vi "Preset_Manager_Main_Integrated2.0.vi"(4 "Virtual Devices List":string[](array[string]), 6 "Filtered Devices List":string[](array[string]), 8 "Experiment Name":string, 10 "DevStatusQueue":refnum<queue>, 11 "Software Root":string) -> ()   [LabVIEW 2020]
uses:
  <vilib>/Utility/miscctls.llb/LVRowAndColumnTypeDef.ctl
  Shared/MySQL/Preset Query Enum.ctl
  <userlib>/_OpenG.lib/array/array.llb/Delete Elements from 1D Array (String)__ogtk.vi
  <userlib>/_OpenG.lib/array/array.llb/openg_array.lvlib
panel:
  out "Queue Progress Bar":ext(slide) scale=0.0..1.0
  out "Queue Size":i32
  out "Current Preset Queue Element":string
  in  "Expt Devices Not On":i32(listbox)
  in  "Preset Devices Not in Experiment":i32(listbox)
  out "Active Preset":string
  out "Preset Execution Indicator":bool caption="Preset Executed"
  in  "EXIT":bool
  in  "Using Queue":bool
  in  "Tab Control":T1(tab)
  in  "Execute Preset":bool
  in  "Delete Preset":bool
  in  "Save as Preset":bool
  in  "Preset Menu":u16(ring) items=["None", "Pulsed Alignment", "3J", "Diode", "26J", "SingleShot", "1Hz", "800 MAX ND", "Amp3-8J-CapExit", "SDI", "CapInHexPosition", "CapOutHexFiberPosition", "Full Heater, Frog Out", "Full Heater, Frog In", "MagSpecSimulateBoff", "Pulsed", "CW", "Amp2, Clunker In", "Amp3-17J", "MagSpecSimulateBon", "SMFiber-In", "SMFiber-Out", "Amp3-MegaAttenuator", "developer", "developer_main", "developer_test_1", "dev_simcam_2", "dev_simcam_3"]
  in  "Load ECS to Table":bool
  in  "Navigate to ECS File":path
  in  "Preset Table Control":string[][](table)
  in  "Choose Values":bool
  in  "Left Join":bool
  in  "Reset Queue":bool
  in  "Queue Table Control":string[][](table)
  in  "Queue Table":string[][](table)
  in  "Execute Queue":bool
  out "PRESET FROM DB":string[][](table)
  out "ECS File":string[][](table)
  out "Coordinate Array":i32[][](array[numeric])
  out "Devices not started":string[](array[string]) caption="Devices not ready for scan"
  out "Active Device array":bool[](array[boolean])
  out "Active Dev/IP":string[](array[string])
  out "Device Errors":string[][](array[string])
  out "Queue Element":i32
  in  "Poll Count":i32
  in  "Mcast address":string
  in  "MCast Remote":u16
  in  "UDP timeout ms":i32
  in  "MC Multicast":refnum<k16>
  in  "My IP":string
  in  "All Devices Core Info":string[][](array[string])
  out "error out":errorcluster
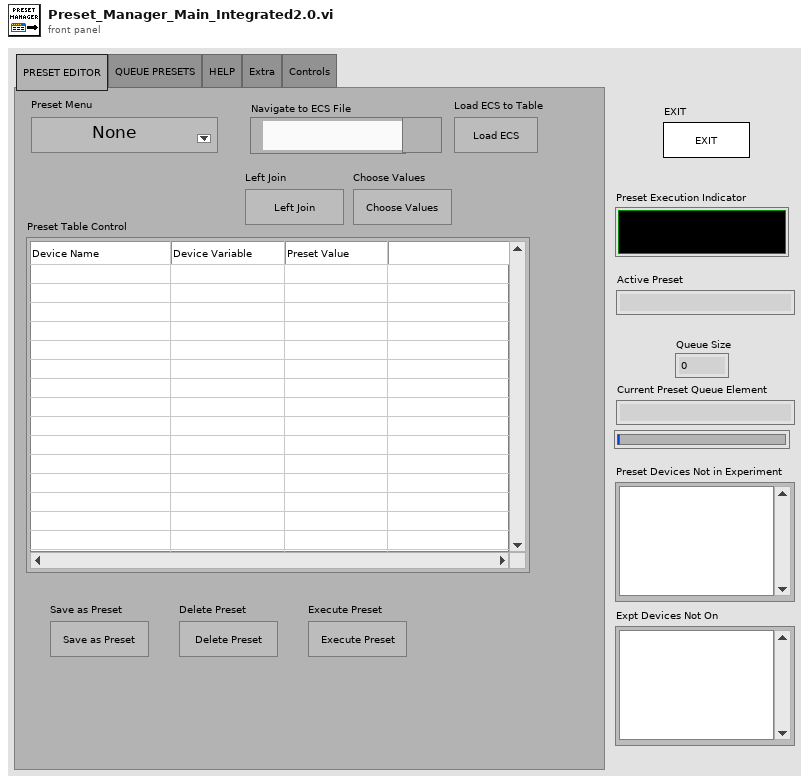
[diagram p1: front panel]
types:
  T1 = enum32{"PRESET EDITOR", "QUEUE PRESETS", "HELP", "Extra", "Controls"}
  T2 = typedef "LVRowAndColumnTypeDef.ctl" = cluster{"Row":i32, "Column":i32}
  T3 = typedef "Preset Query Enum.ctl" = enum16{"Get Locations", "Get all IPs and MACs", "Get classes", "Get expt variables to set at scanstart for particular device", "Get expt devices and variables with start values", "Get expt devices and variables (with data to get)", "Get expt devices with data to get", "Get Expt devices and GUIs", "Get all devices basic properties", "Get Virtual Devices Core Info", "Get Expt names", "Get experiment basic properties", "Get experiment alarm variables", "Get MC Ports", "Get device network comm port", "Get devicetype lvclass path", "Get basic device properties", "Get Init Order", "Get all setable variables of a device", "Get device variable aliases", "Get force values of all settable variables", "Get all variables of a devicetype", "Get all variables of a device", "Get plotter details", "Get Saved Scans", "Get Scan Info", "GetGeneralGUIs", "Get expt for plotter", "Get plotter IDs from expt", "Get all devices", "Get all Virtual Devices", "Get all aliases", "Get variable and device info for Virtual Device", "GetItemLocatorIP", "Get IPs for GUIs", "Get DeviceType from Device", "GetLocalPortRange", "GetDevicePresetVariables", "Get Device Configuration", "GetAllPresetNames", "GetAllConfigurationNames", "GetPresetDeviceNames", "GetDeviceAliases", "GetDevicesOfClass"}
  T4 = enum32{"Invalid", "Standard", "Closed", "Hidden", "Minimized", "Maximized"}
  T5 = enum32{"invalid app kind", "Development System", "Run Time System", "Student Edition", "Embedded LabVIEW", "Evaluation", "Custom"}
  T6 = cluster{"Core":cluster{"Current VI Reference":refnum<vi>, "Close Panel on Exit?":bool}, "Your Boolean data":bool, "String":string, "Preset Table Control":string[][], "Column Headers[]":string[], "Queue Table Control":string[][], "Preset Manager Cluster":cluster{"PresetName":string, "Mcast command":string, "Current Preset Devices":string[], "My IP":string, "Mcast address":string, "Software Root":string, "Experiment Name":string, "MCast Remote":u16, "UDP timeout ms":i32, "MC Multicast":refnum<k16>, "All Devices Core Info":string[][], "Filtered Devices List":string[], "Virtual Devices List":string[], "DevStatusQueue":refnum<queue>}}
  T7 = typedef "LVPoint32TypeDef.ctl" = cluster{"Horizontal":i32, "Vertical":i32}
  T8 = cluster{"Current VI Reference":refnum<vi>, "Close Panel on Exit?":bool}
  T9 = cluster{"PresetName":string, "Mcast command":string, "Current Preset Devices":string[], "My IP":string, "Mcast address":string, "Software Root":string, "Experiment Name":string, "MCast Remote":u16, "UDP timeout ms":i32, "MC Multicast":refnum<k16>, "All Devices Core Info":string[][], "Filtered Devices List":string[], "Virtual Devices List":string[], "DevStatusQueue":refnum<queue>}
  T10 = enum16{"Left Button", "Center Button", "Right Button", "Window Close"}
  T11 = typedef "mysql_authentication.ctl" = cluster{"User":string, "Password":string, "Database":string}
  T12 = cluster{"Port":u16, "IP Address":string, "Authentication":T11}
  T13 = typedef "preset diagnostics.ctl" = cluster{"Active Preset Achieved":bool, "Devices with Active Preset Not Set":string[], "Dev Presets":string[], "All Preset Devices ON?":bool[]}
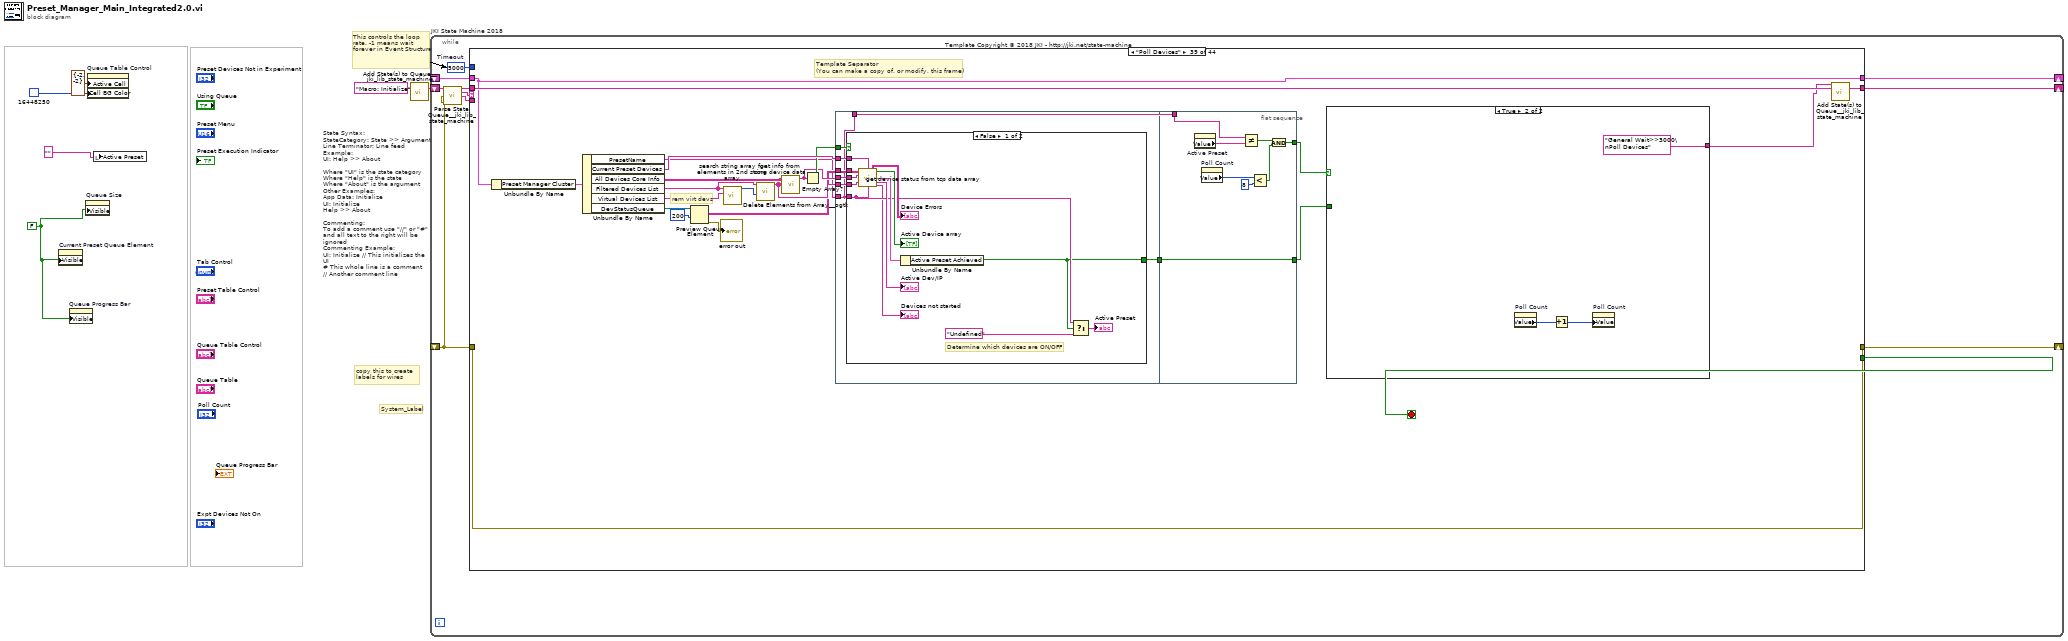
[diagram p0: block diagram]
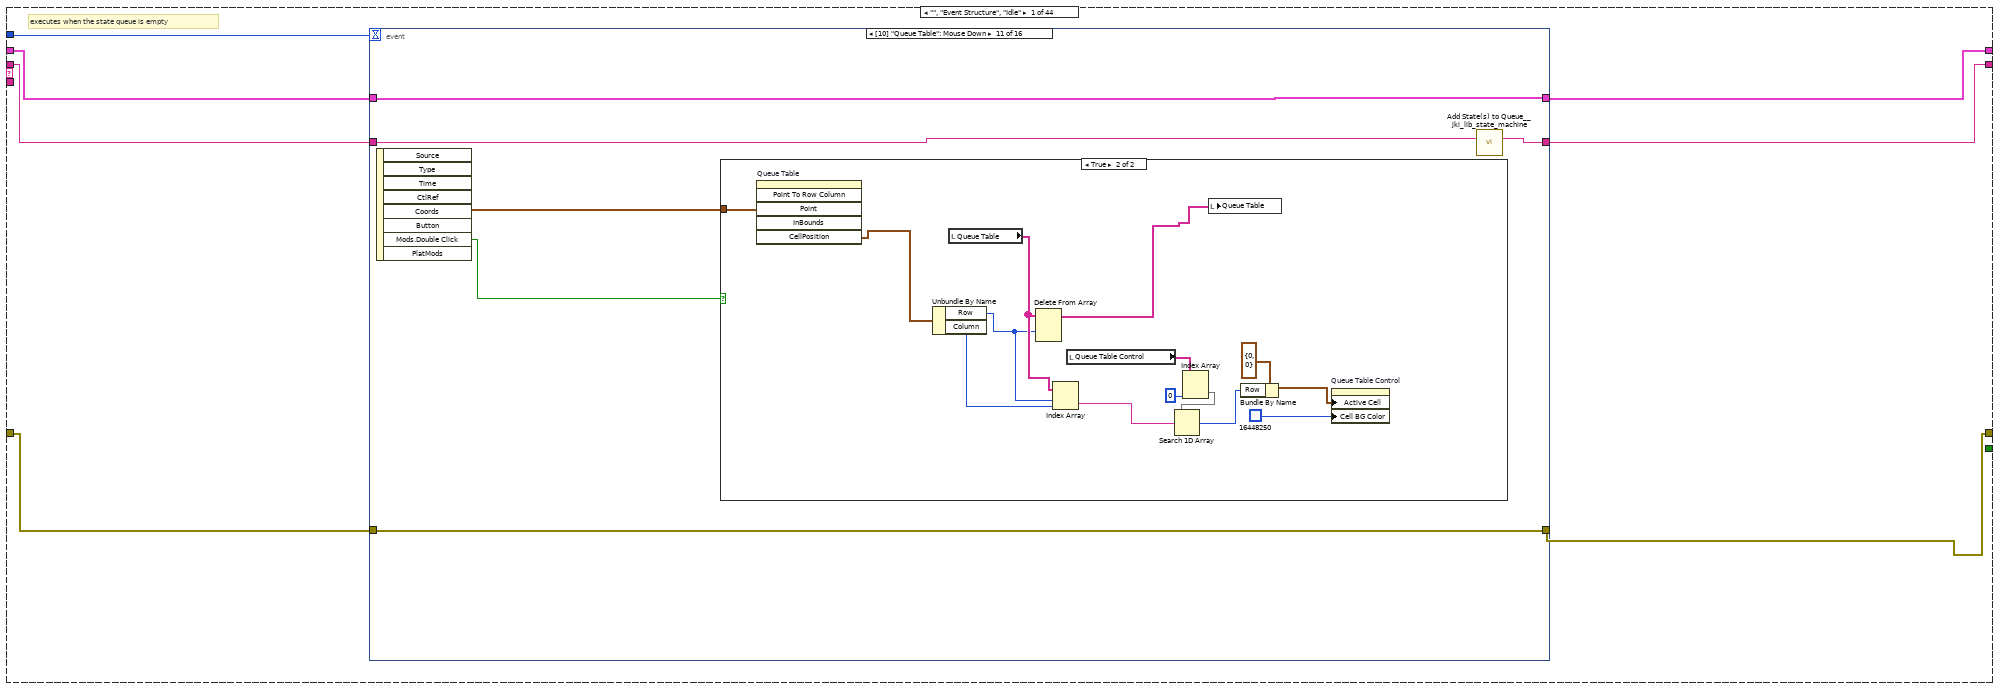
[diagram p2: hidden frame]
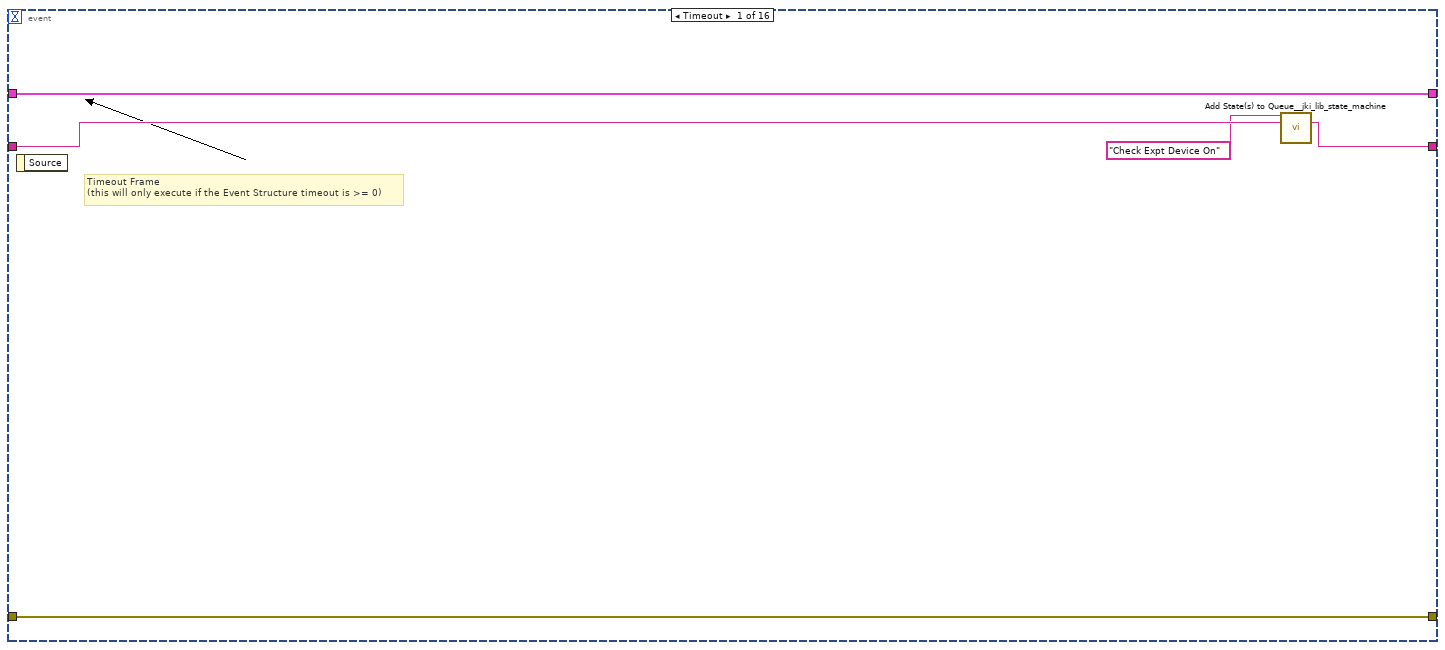
[diagram p3: hidden frame]
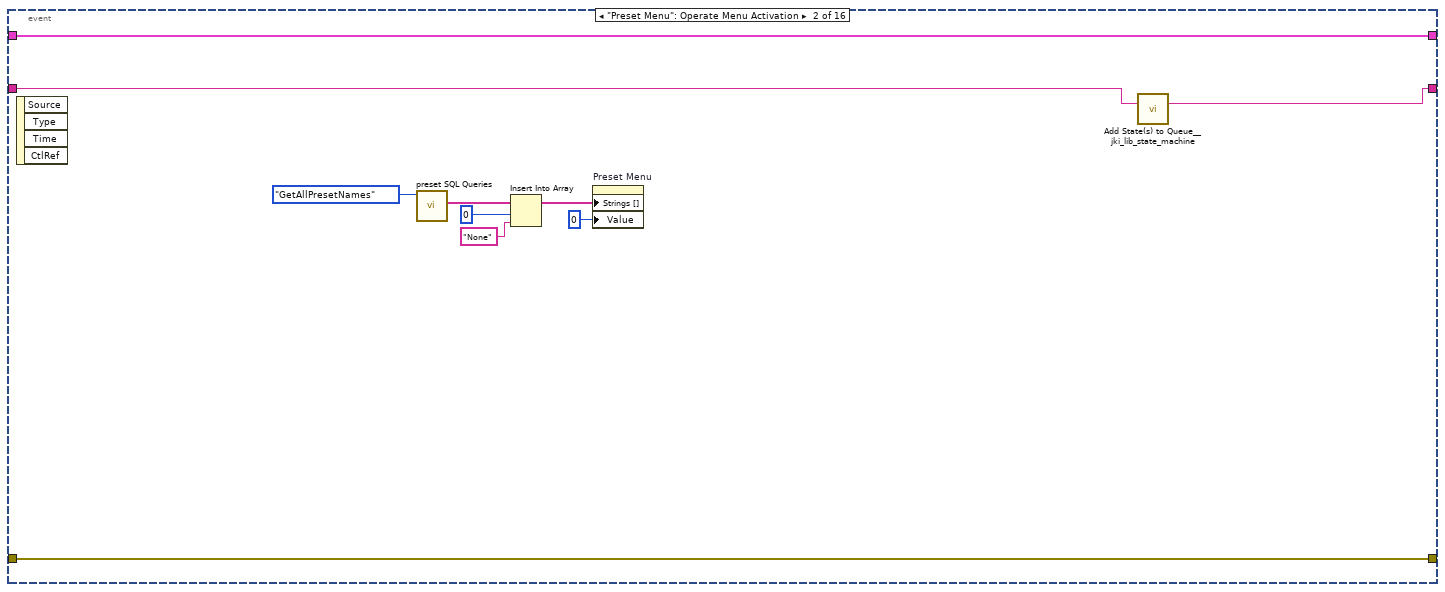
[diagram p4: hidden frame]
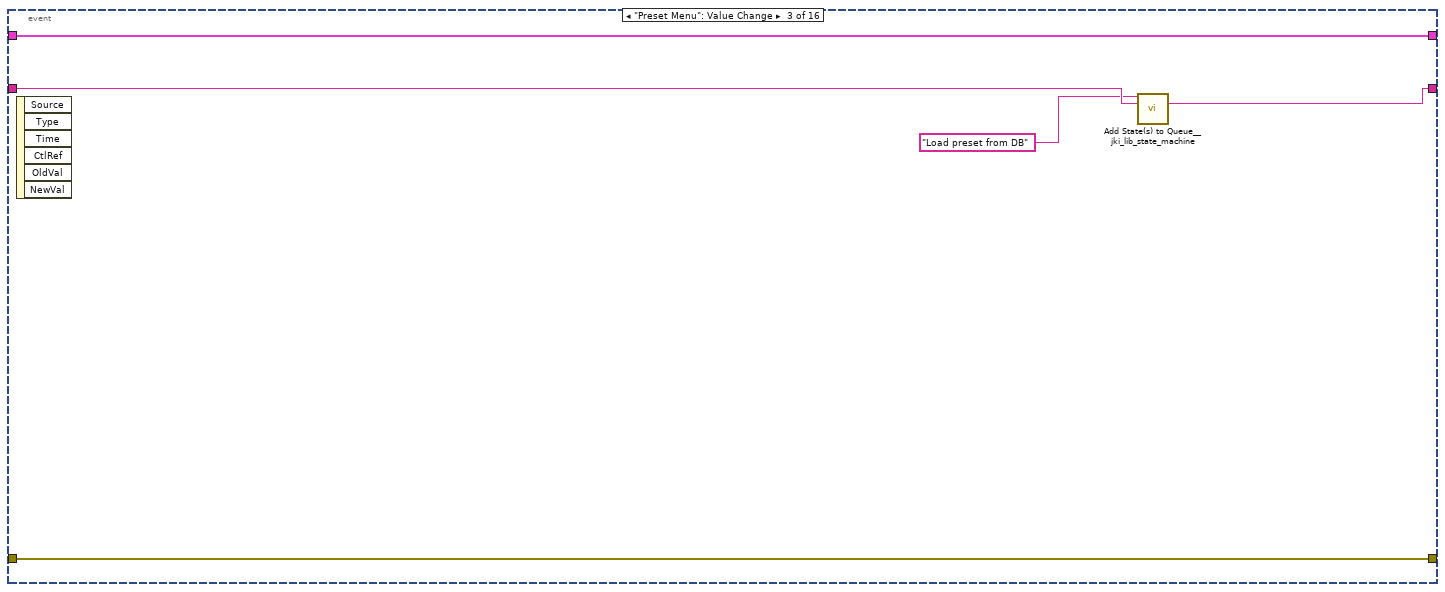
[diagram p5: hidden frame]
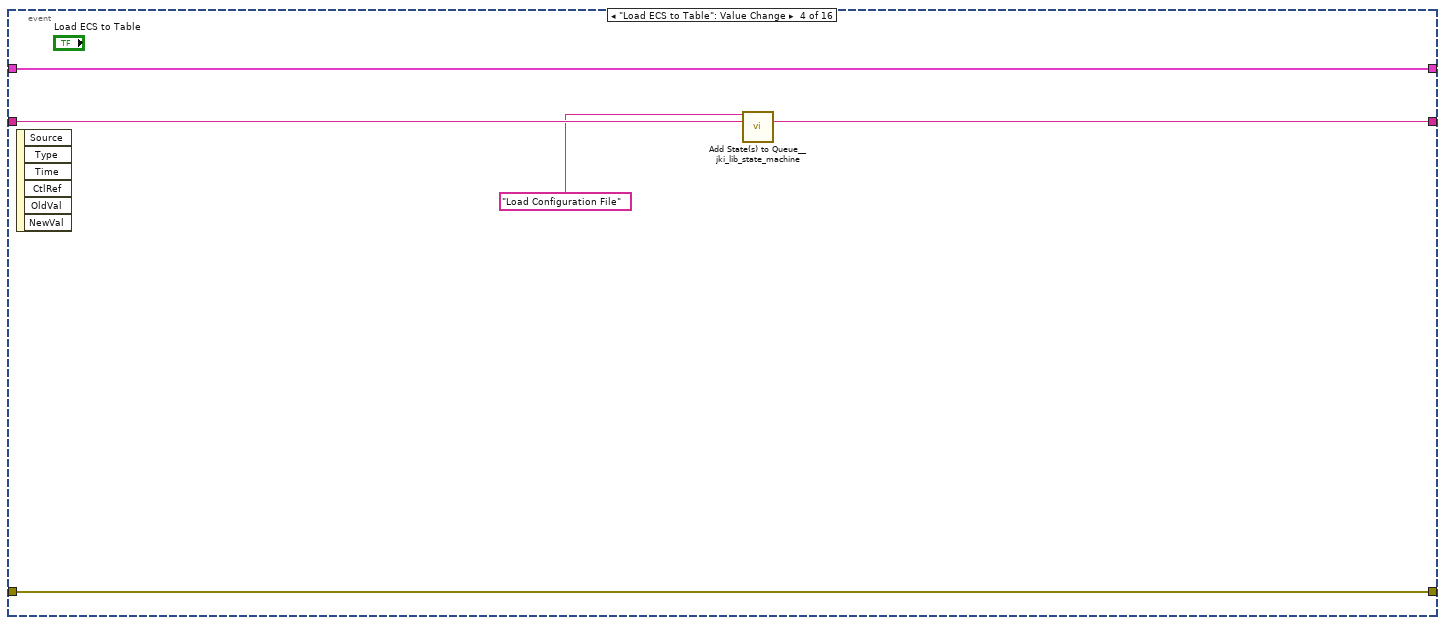
[diagram p6: hidden frame]
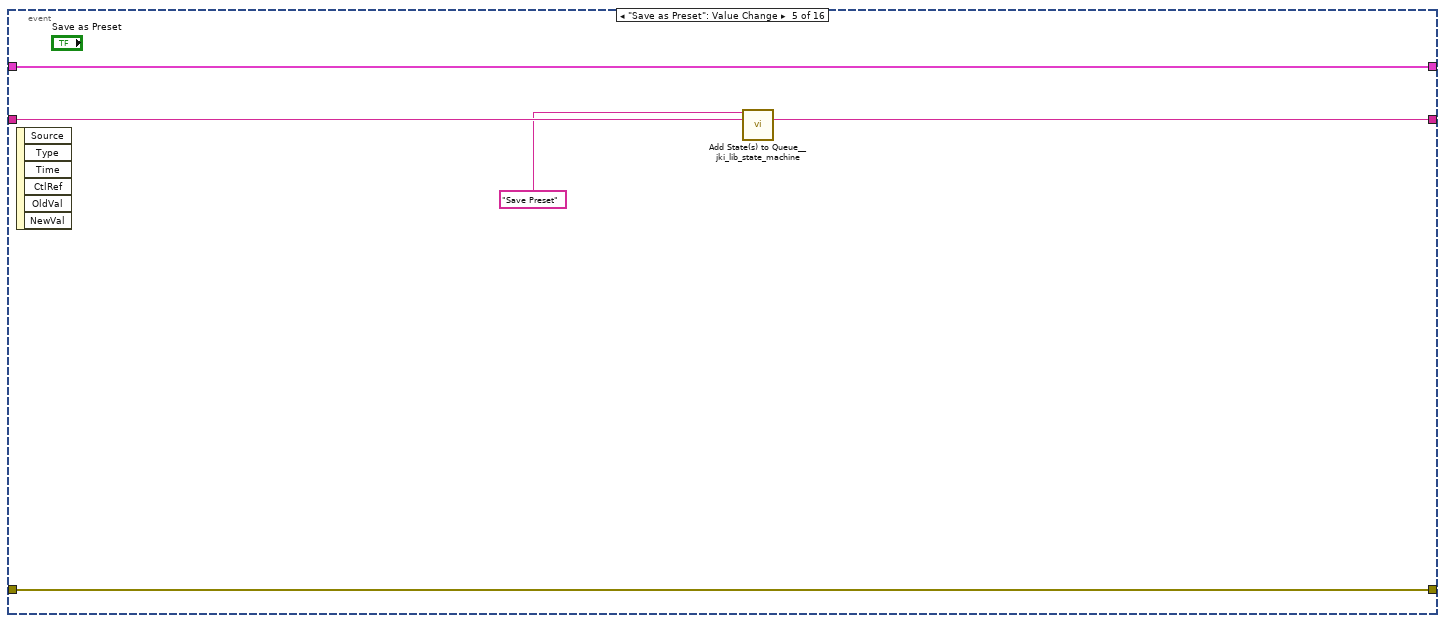
[diagram p7: hidden frame]
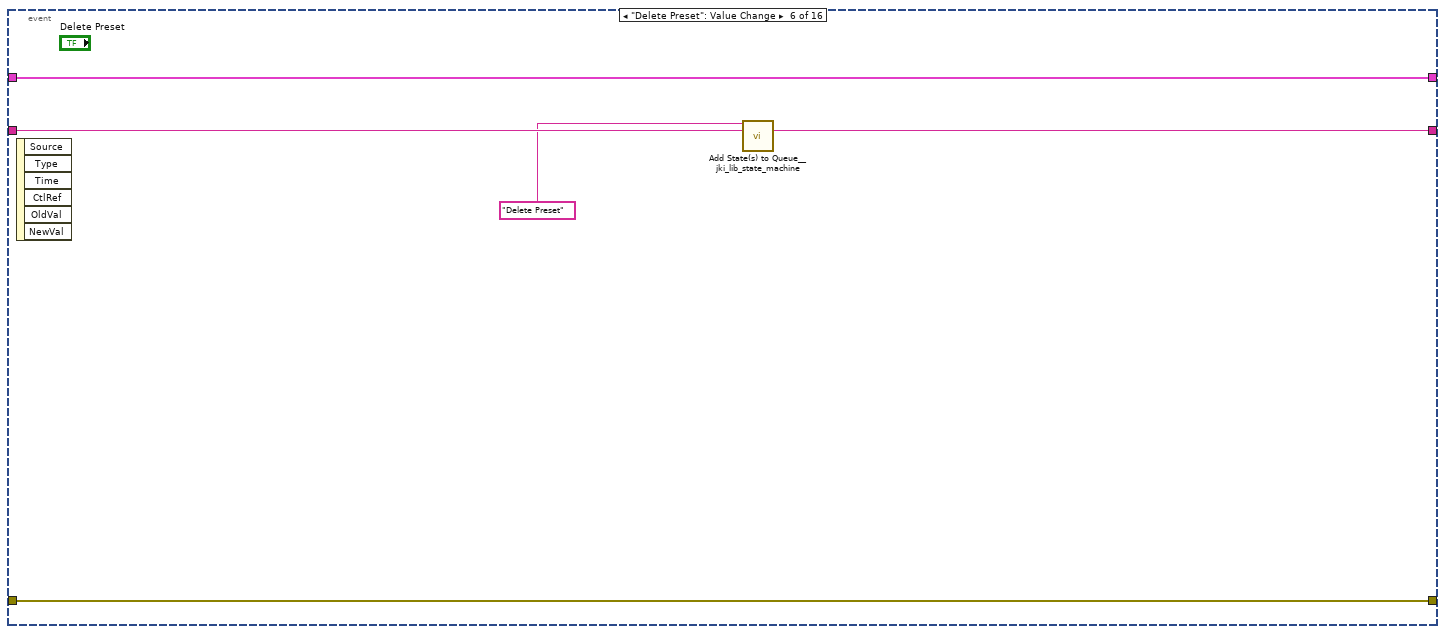
[diagram p8: hidden frame]
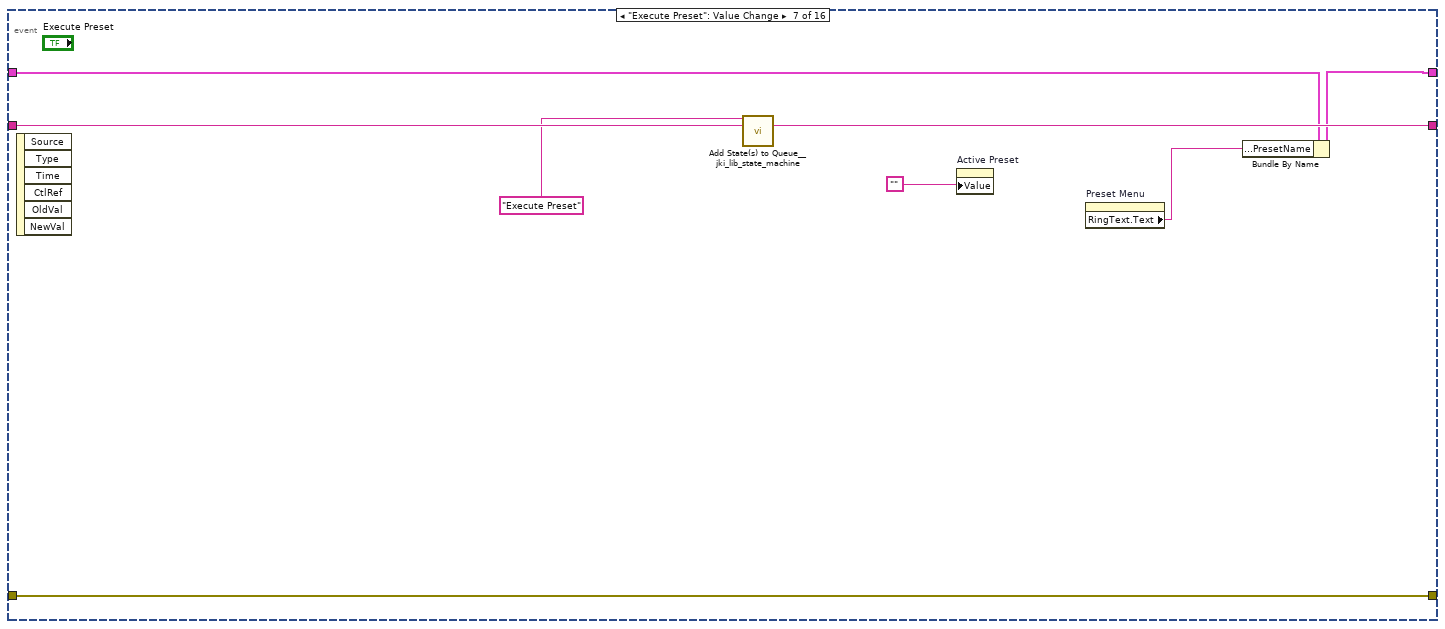
[diagram p9: hidden frame]
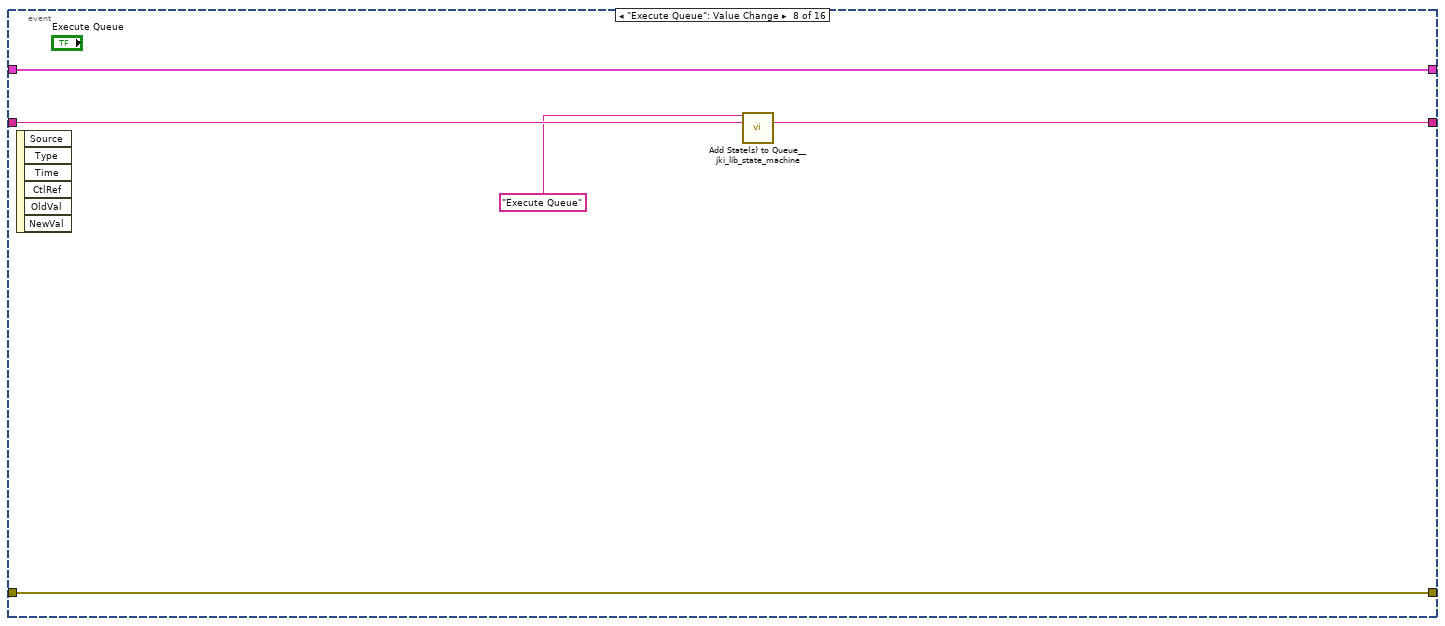
[diagram p10: hidden frame]
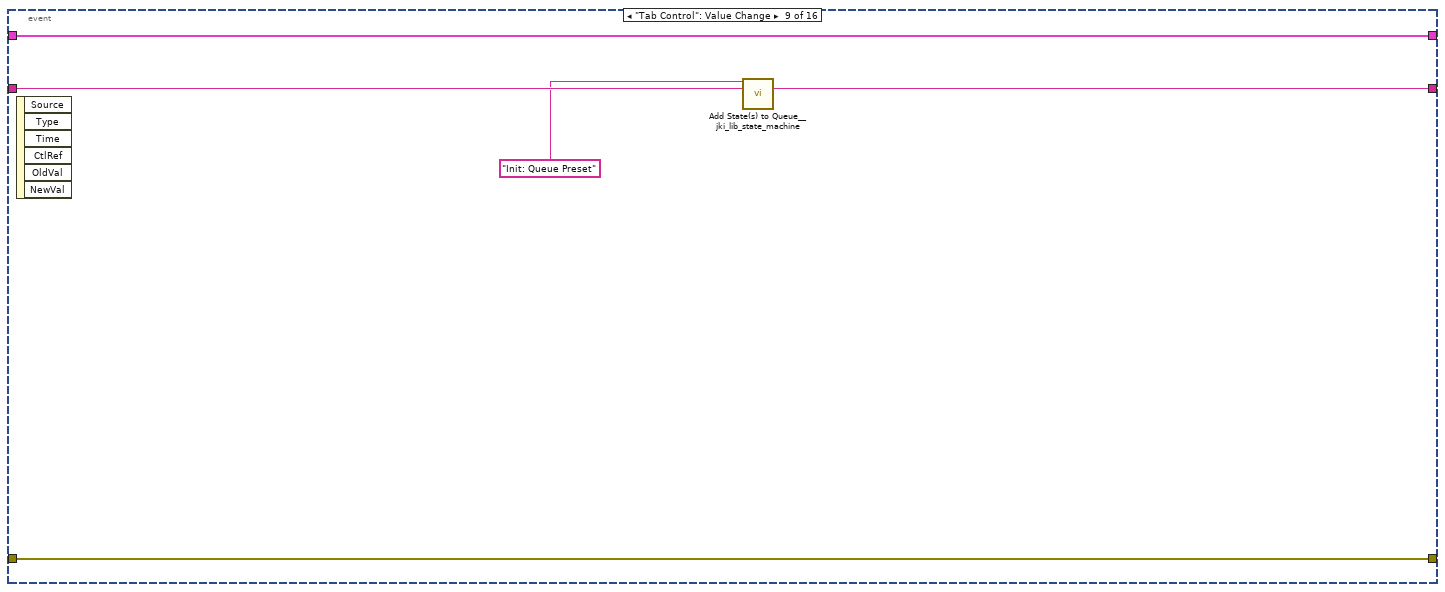
[diagram p11: hidden frame]
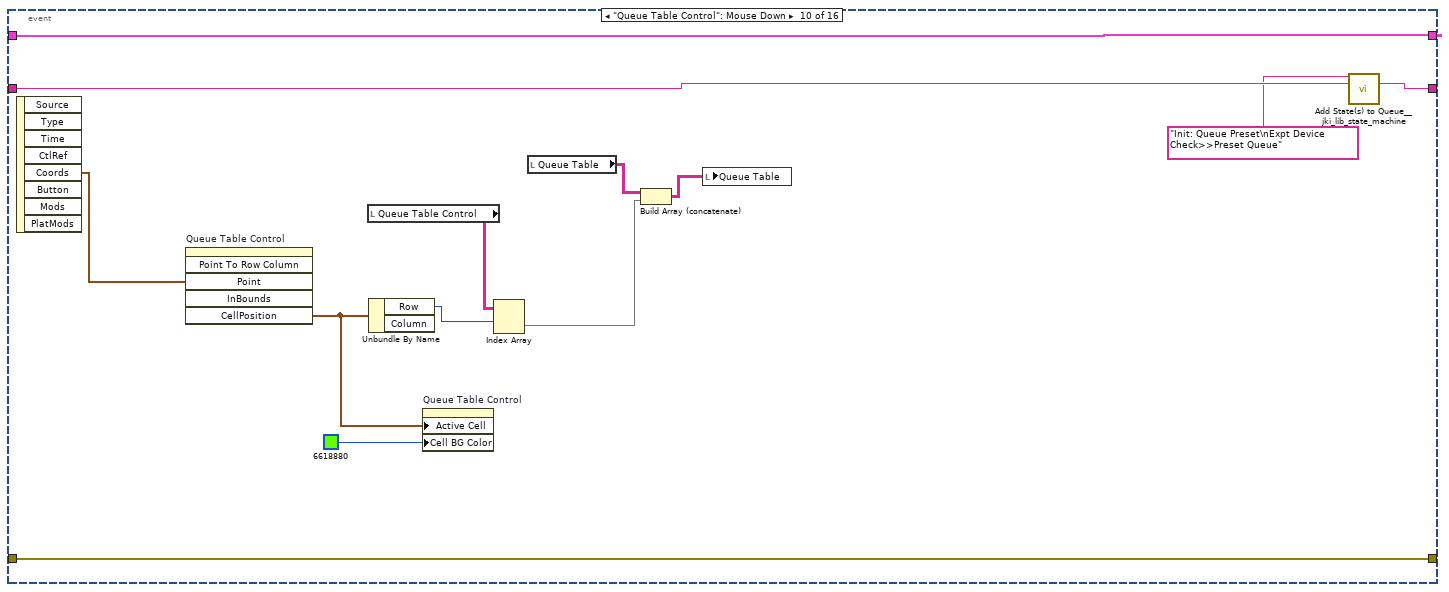
[diagram p12: hidden frame]
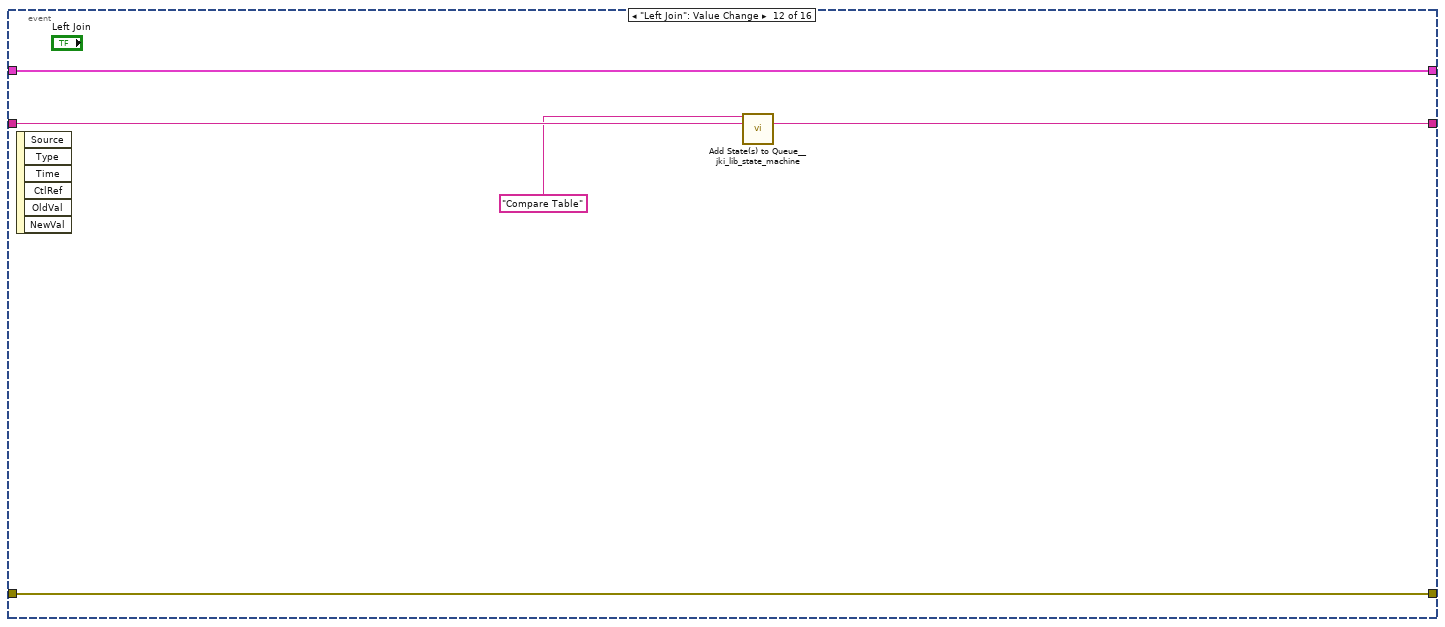
[diagram p14: hidden frame]
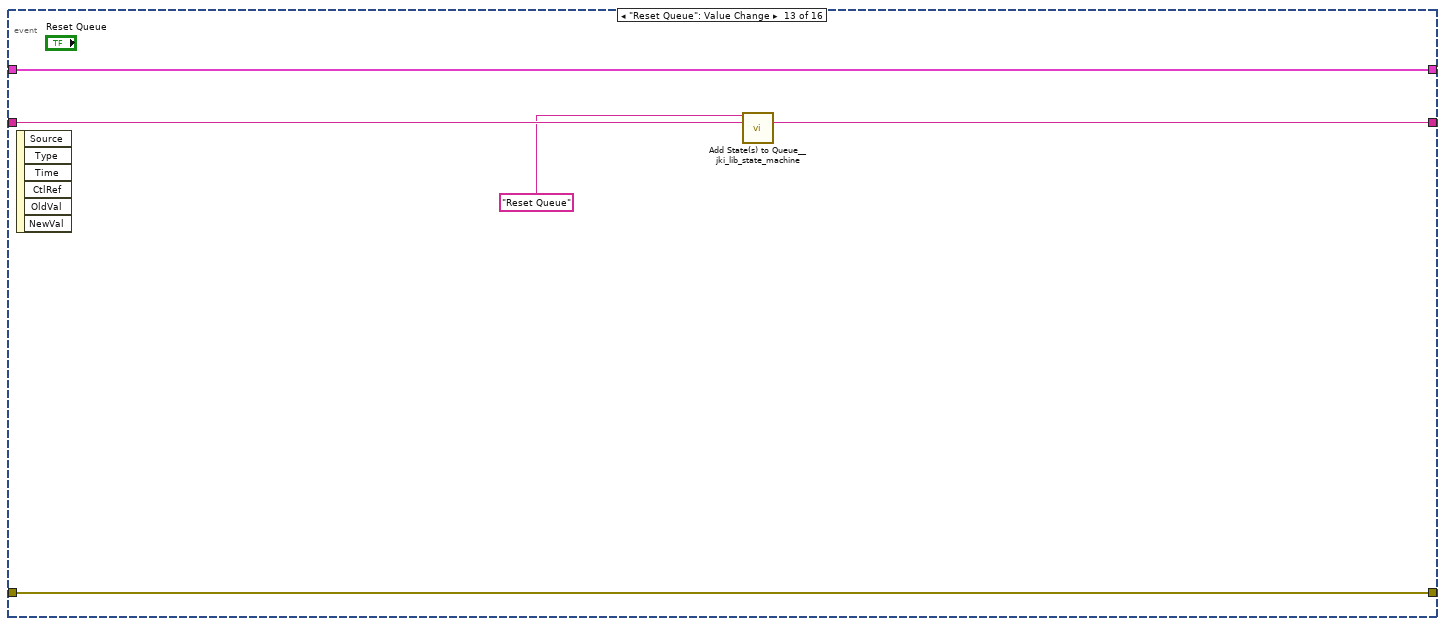
[diagram p15: hidden frame]
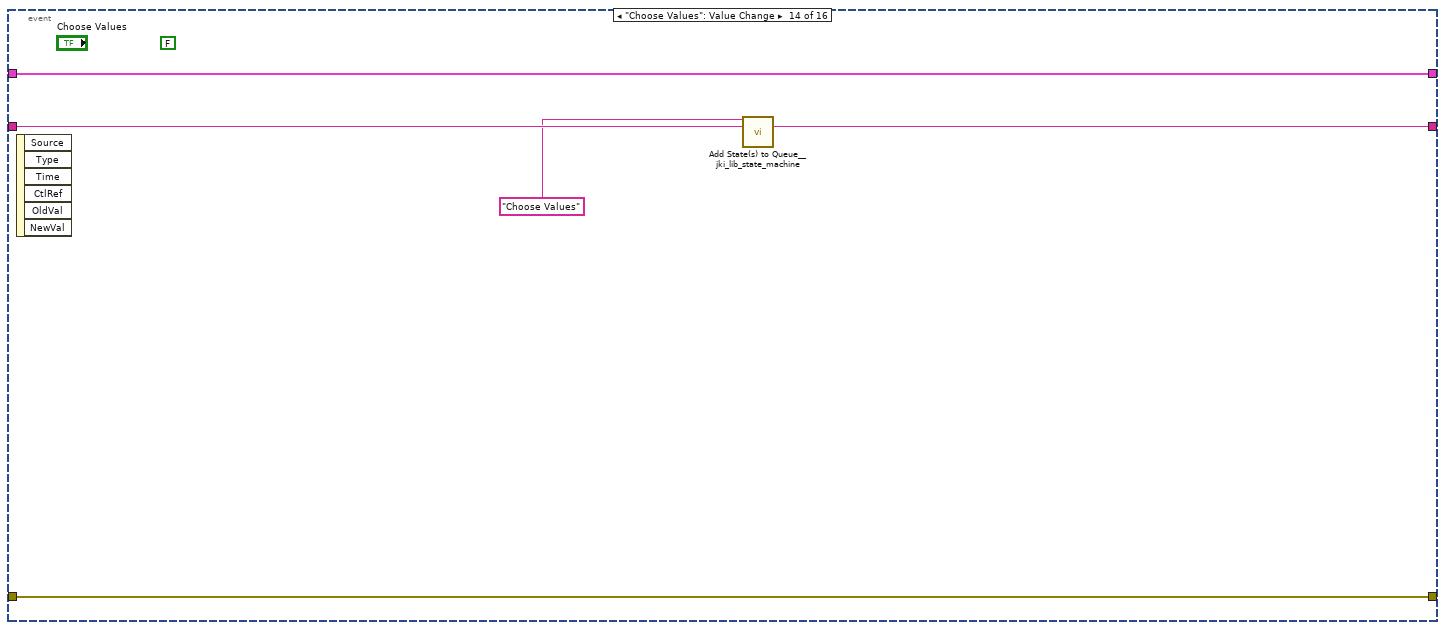
[diagram p16: hidden frame]
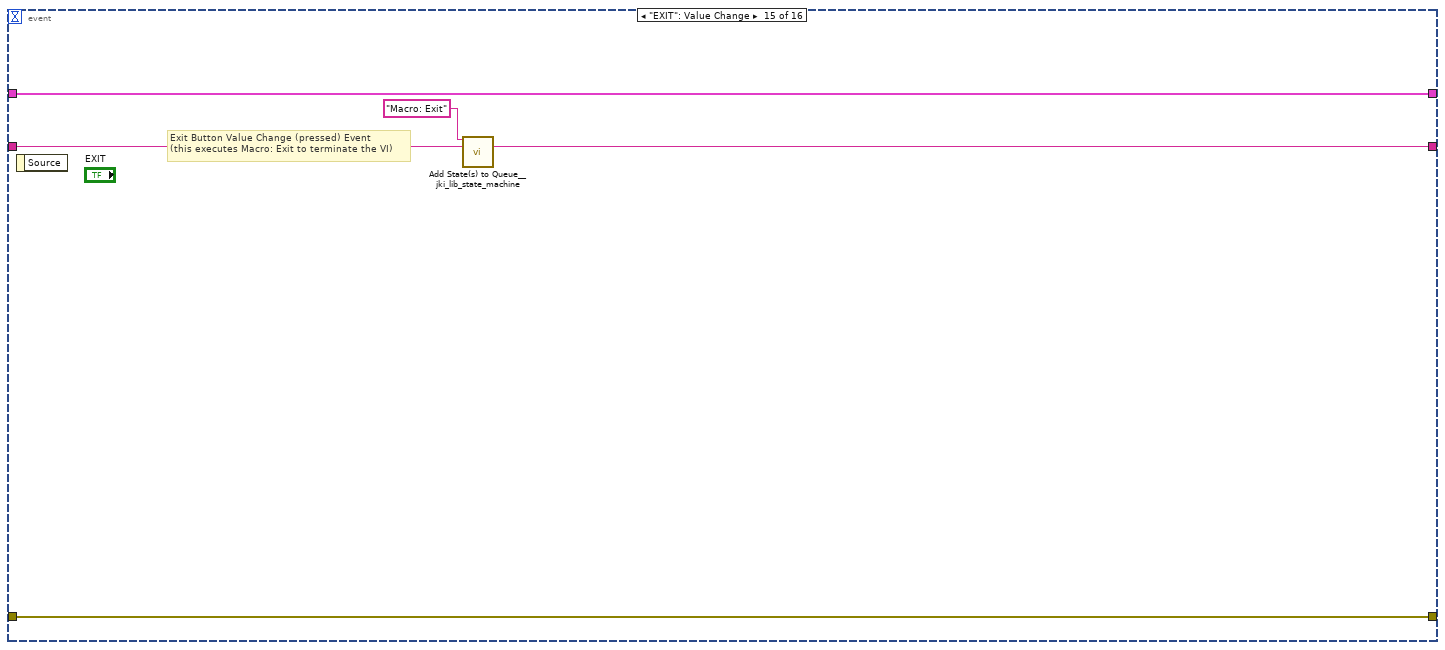
[diagram p17: hidden frame]
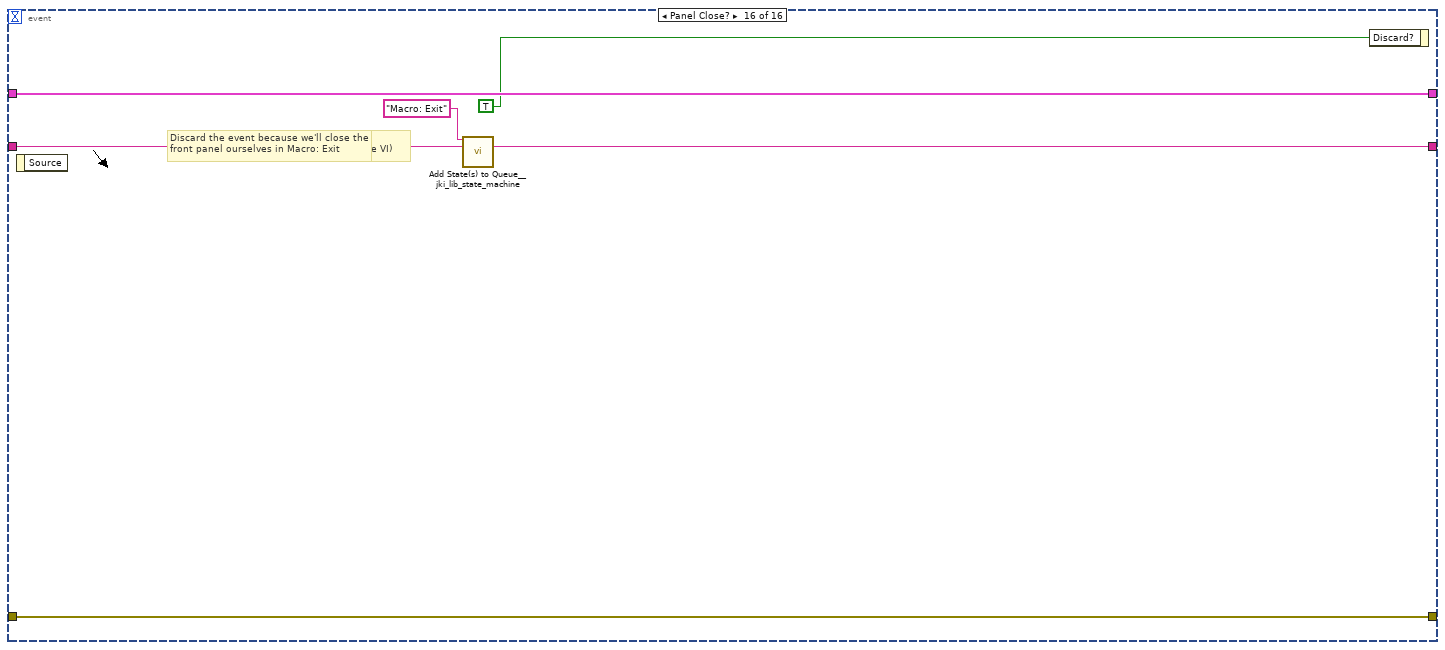
[diagram p18: hidden frame]
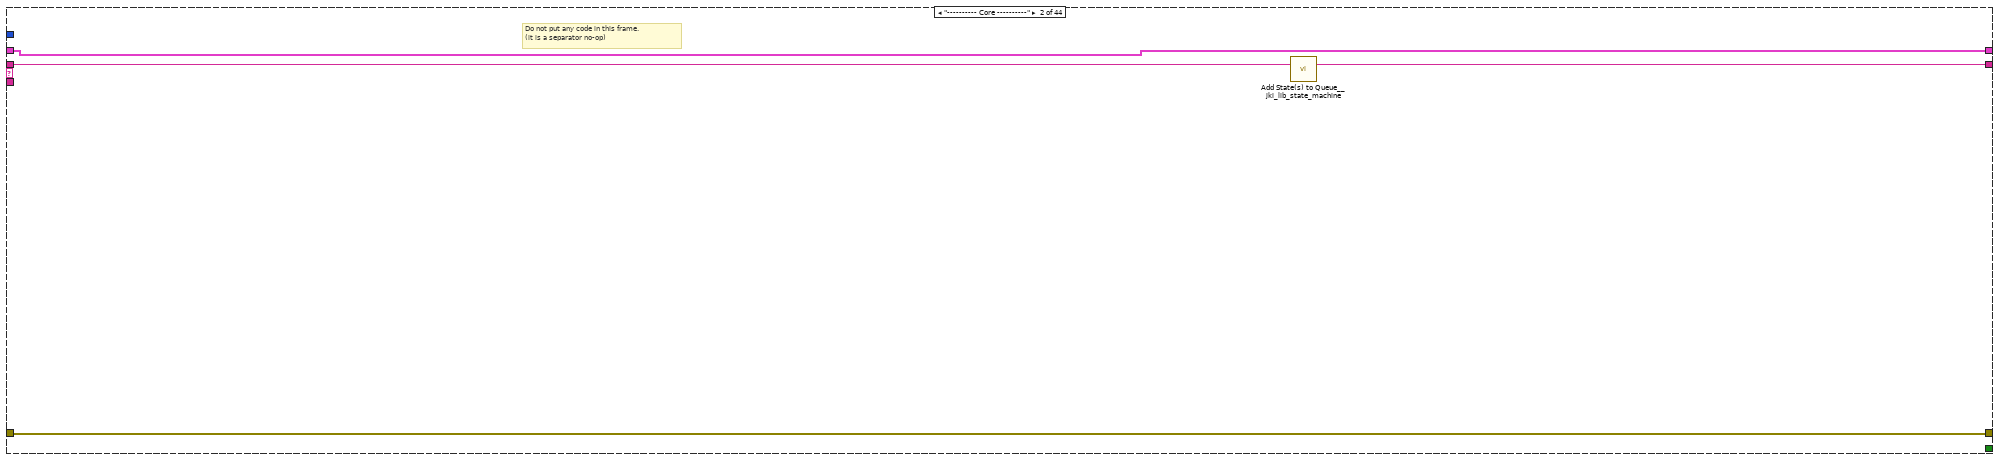
[diagram p19: hidden frame]
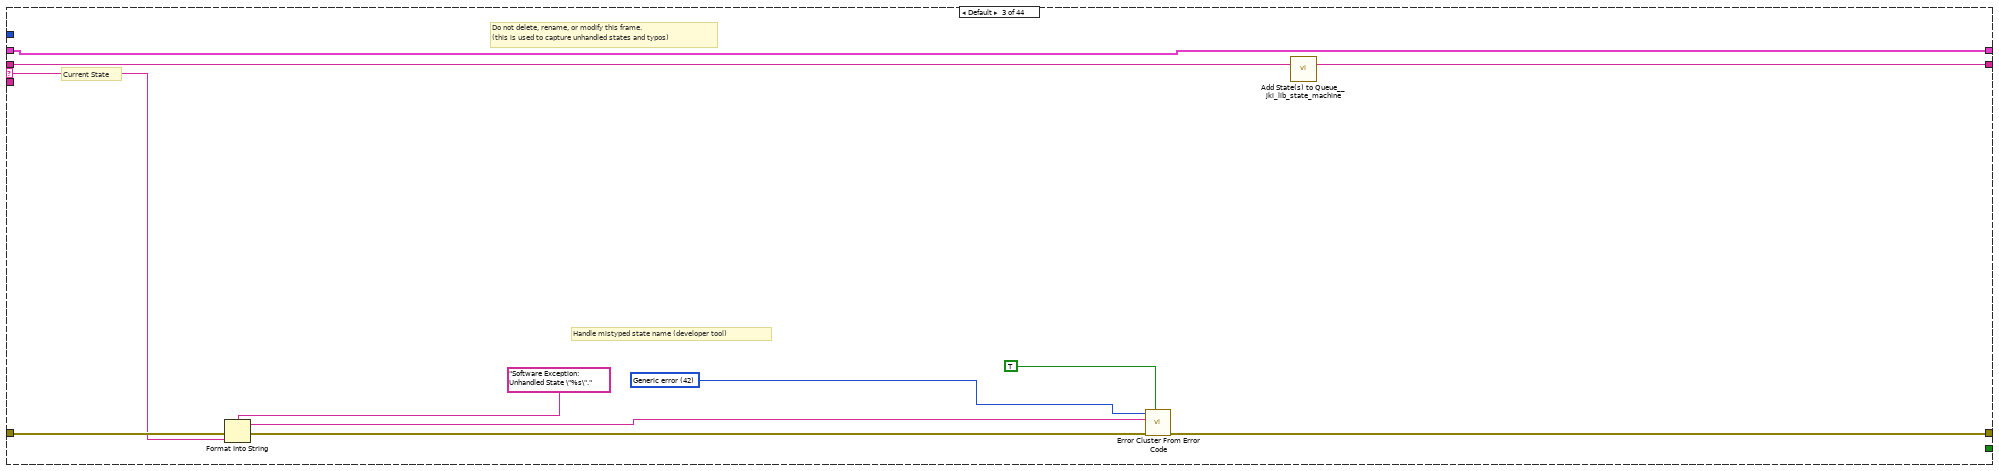
[diagram p20: hidden frame]
diagram:
  w1 = FALSE
  # "State Syntax:\nStateCategory: State >> Argument\nLine Terminator: Line feed\nExample:\nUI: Help >> About\n\nWhere \"UI\" is the state category\nWhere \"Help\" is the state\nWhere \"About\" is the argument\nOther Examples:\nApp Data: Initialize\nUI: Initialize\nHelp >> About\n\nCommenting:\nTo add a comment use \"//\" or \"#\" and all text to the right will be ignored\nCommenting Example:\nUI: Initialize // This initializes the UI\n# This whole line is a comment\n// Another comment line"
  # "copy this to create labels for wires"
  # "This controls the loop rate. -1 means wait forever in Event Structure"
  # "System_Label"
  n1 = property on="Current Preset Queue Element" class="Str"("Visible"=w1) -> ()  [unwired: 2 in, 2 out]
  n2 = property on="Queue Progress Bar" class="Slide (strict)"("Visible"=w1) -> ()  [unwired: 2 in, 2 out]
  n3 = property on="Queue Size" class="DigNum (strict)"("Visible"=w1) -> ()  [unwired: 2 in, 2 out]
  n4 = property on="Queue Table Control" class="Tbl (strict)"("Active Cell"=T2 {"Row"=-2, "Column"=-2} ("Active Cell:Active Cell"), "Cell BG Color"=u32 16448250 ("Active Cell:Cell Background Color")) -> ()  [unwired: 2 in, 2 out]
  n5 = local write "Active Preset"("" ("My IP")) -> ()
  n6 = call <vilib>:"Add State(s) to Queue__jki_lib_state_machine.vi"("State(s) in (\"\")"="Macro: Initialize") -> ("States Out"=w6:string)  [unwired: 14 in]
  n7 = while "JKI State Machine 2018" {
    shift-right: [w7] -> _
    shift-left: _ -> [w10]
    shift-right: [w13] -> _
    shift-left: _ -> [w8]
    shift-right: [w12] -> _
    shift-left: w6 -> [w14]
    stop <- w11 stop-if-true
    w9 = 5000  # Timeout
    # "Template Copyright © 2018 JKI - http://jki.net/state-machine"
    n8 = call <vilib>:"Parse State Queue__jki_lib_state_machine.vi"("State Queue"=w14, "Error In (no error)"=w8) -> ("Remaining States"=w16:string, "Current State"=w17:string, "Arguments"=w15:string)  [unwired: 11 in]
    n9 = case shown="\"Poll Devices\"" w17 {
      selector: w17 -> [_ _ w141 _ _ _ _ _ _ _ _ _ _ _ _ _ _ _ _ _ _ _ _ _ _ _ _ _ _ _ _ _ _ _ _ _ _ _ _ _ _ _ _ _]
      tunnel: w16 -> [w24 w140 w145 w164 w170 w175 w179 w196 w202 w206 w210 w216 w227 w296 w307 w317 w329 w333 w343 w351 w361 w370 w379 w389 w406 w432 w466 w480 w484 w490 w494 w501 w510 w515 w530 w557 w562 w578 w601 w664 w676 w680 w697 w713]
      tunnel: w15 -> [_ _ _ _ _ _ _ _ _ _ _ w211 w221 _ _ _ _ _ _ _ _ _ _ _ _ _ _ _ _ _ _ _ _ _ _ _ _ w572 _ _ _ _ w688 _]
      tunnel: w10 -> [w22 w137 w143 w157 w167 w173 w176 _ w197 w203 w208 w214 w223 w293 w304 w314 w326 w330 w338 w344 w357 w367 w375 w386 w403 w429 w462 w476 w481 w487 w491 w496 w507 w511 w526 w554 w559 w575 w597 w657 w667 w677 w694 w710]
      tunnel: [w21 w138 w147 w161 errorcluster {"status"=FALSE, "code"=0, "source"=""} ("error out") w172 w177 w194 w198 w204 w207 w212 w224 w294 w305 w315 w327 w331 w341 w349 w359 w368 w377 w387 w404 w430 w464 w478 w482 w488 w492 w499 w508 w513 w528 w555 w560 w576 w599 w662 w674 w678 w695 w711] -> w13
      tunnel: w8 -> [w20 w138 w146 w161 w166 w172 w177 w194 w199 w204 w207 w213 w225 w294 w305 w315 w327 w331 w341 w349 w359 w368 w377 w387 w404 w430 w464 w478 w482 w488 w492 w499 w508 w513 w528 w555 w560 w576 w599 w662 w674 w678 w695 w711]
      tunnel: [w23 w139 w144 w163 w169 w174 w178 w195 w201 w205 w209 w215 w226 w295 w306 w316 w328 w332 w342 w350 w360 w369 w378 w388 w405 w431 w465 w479 w483 w489 w493 w500 w509 w514 w529 w556 w561 w577 w600 w663 w675 w679 w696 w712] -> w12
      tunnel: [_ _ _ _ _ TRUE _ _ _ _ _ _ _ _ _ _ _ _ _ _ _ _ _ _ _ _ _ _ _ _ _ _ _ _ _ _ _ _ _ _ _ _ _ _] -> w11
      tunnel: w9 -> [w18 _ _ _ _ _ _ _ _ _ _ _ _ _ _ _ _ _ _ _ _ _ _ _ _ _ _ _ _ _ _ _ _ _ _ _ _ _ _ _ _ _ _ _]
      tunnel: [w19 w137 w143 w162 w167 w173 w176 w185 w197 w203 w208 w214 w223 w293 w304 w314 w325 w330 w336 w344 w356 w366 w374 w386 w403 w429 w462 w476 w481 w487 w491 w496 w507 w511 w525 w554 w558 w575 w597 w658 w666 w677 w694 w710] -> w7
      frame "", "Event Structure", "Idle" {
        # "executes when the state queue is empty"
        n10 = event shown="[10] \"Queue Table\": Mouse Down" {
          selector: _ -> [_ _ _ _ _ _ _ _ _ _ _ _ _ _ _ _]
          dyn-events: _ -> [_ _ _ _ _ _ _ _ _ _ _ _ _ _ _ _]
          timeout: w18 -> [_ _ _ _ _ _ _ _ _ _ _ _ _ _ _ _]
          tunnel: w24 -> [w29 w31 w42 w47 w52 w57 w66 w70 w76 w89 w95 w113 w118 w123 w130 w136]
          tunnel: [w28 w30 w41 w46 w51 w56 w65 w69 w75 w88 w94 w112 w117 w122 w129 w135] -> w23
          tunnel: w22 -> [w26 w39 w44 w49 w54 w59 w61 w72 w73 w86 w93 w115 w120 w125 w127 w133]
          tunnel: [w27 w38 w43 w48 w53 w58 w67 w71 w77 w90 w96 w114 w119 w124 w128 w134] -> w21
          tunnel: w20 -> [w27 w38 w43 w48 w53 w58 w67 w71 w77 w90 w96 w114 w119 w124 w128 w134]
          tunnel: [w26 w39 w44 w49 w54 w59 w60 w72 w73 w86 w93 w115 w120 w125 w127 w133] -> w19
          event Timeout {
            # "Timeout Frame\n(this will only execute if the Event Structure timeout is >= 0)"
            n11 = event-data() -> ()  [unwired: 1 in, 1 out]
            n12 = call <vilib>:"Add State(s) to Queue__jki_lib_state_machine.vi"("State(s) in Front (\"\")"="Check Expt Device On" ("State(s) in Front (\"\")"), "State(s) in (\"\")"=w29) -> ("States Out"=w28:string)  [unwired: 13 in]
          }
          event "Preset Menu": Operate Menu Activation {
            n13 = event-data() -> ()  [unwired: 1 in, 4 out]
            n14 = call "preset SQL Queries.vi"("Preset Query"=Preset_Query_Enum."GetAllPresetNames") -> ("1st column 1st data"=w36:string[])  [unwired: 8 in, 2 out]
            n15 = Insert Into Array(array=w36, index=0, new element="None" ("new element/subarray")) -> (w33:string[])
            n16 = property on="Preset Menu" class="Ring (strict)"("Strings []"=w33, "Value"=0 ("index")) -> ()  [unwired: 2 in, 2 out]
            n17 = call <vilib>:"Add State(s) to Queue__jki_lib_state_machine.vi"("State(s) in (\"\")"=w31) -> ("States Out"=w30:string)  [unwired: 14 in]
          }
          event "Preset Menu": Value Change {
            n18 = event-data() -> ()  [unwired: 1 in, 6 out]
            n19 = call <vilib>:"Add State(s) to Queue__jki_lib_state_machine.vi"("State(s) in Front (\"\")"="Load preset from DB" ("State(s) in Front (\"\")"), "State(s) in (\"\")"=w42) -> ("States Out"=w41:string)  [unwired: 13 in]
          }
          event "Load ECS to Table": Value Change {
            n20 = event-data() -> ()  [unwired: 1 in, 6 out]
            n21 = call <vilib>:"Add State(s) to Queue__jki_lib_state_machine.vi"("State(s) in Front (\"\")"="Load Configuration File", "State(s) in (\"\")"=w47) -> ("States Out"=w46:string)  [unwired: 13 in]
          }
          event "Save as Preset": Value Change {
            n22 = event-data() -> ()  [unwired: 1 in, 6 out]
            n23 = call <vilib>:"Add State(s) to Queue__jki_lib_state_machine.vi"("State(s) in Front (\"\")"="Save Preset", "State(s) in (\"\")"=w52) -> ("States Out"=w51:string)  [unwired: 13 in]
          }
          event "Delete Preset": Value Change {
            n24 = event-data() -> ()  [unwired: 1 in, 6 out]
            n25 = call <vilib>:"Add State(s) to Queue__jki_lib_state_machine.vi"("State(s) in Front (\"\")"="Delete Preset", "State(s) in (\"\")"=w57) -> ("States Out"=w56:string)  [unwired: 13 in]
          }
          event "Execute Preset": Value Change {
            n26 = event-data() -> ()  [unwired: 1 in, 6 out]
            n27 = call <vilib>:"Add State(s) to Queue__jki_lib_state_machine.vi"("State(s) in Front (\"\")"="Execute Preset", "State(s) in (\"\")"=w66) -> ("States Out"=w65:string)  [unwired: 13 in]
            n28 = property on="Active Preset" class="Str"("Value"="") -> ()  [unwired: 2 in, 2 out]
            n29 = property on="Preset Menu" class="Ring (strict)"() -> ("RingText.Text"=w62:string)  [unwired: 2 in, 2 out]
            n30 = Bundle By Name(cluster=w61, "Preset Manager Cluster.PresetName"=w62) -> (w60:T6)
          }
          event "Execute Queue": Value Change {
            n31 = event-data() -> ()  [unwired: 1 in, 6 out]
            n32 = call <vilib>:"Add State(s) to Queue__jki_lib_state_machine.vi"("State(s) in Front (\"\")"="Execute Queue", "State(s) in (\"\")"=w70) -> ("States Out"=w69:string)  [unwired: 13 in]
          }
          event "Tab Control": Value Change {
            n33 = event-data() -> ()  [unwired: 1 in, 6 out]
            n34 = call <vilib>:"Add State(s) to Queue__jki_lib_state_machine.vi"("State(s) in Front (\"\")"="Init: Queue Preset", "State(s) in (\"\")"=w76) -> ("States Out"=w75:string)  [unwired: 13 in]
          }
          event "Queue Table Control": Mouse Down {
            n35 = event-data() -> ("Coords"=w85:T7)  [unwired: 1 in, 7 out]
            n36 = invoke on="Queue Table Control" class="Tbl (strict)" method="Point To Row Column"("Point"=w85) -> ("CellPosition"=w82:T2)  [unwired: 5 in, 5 out]
            n37 = local read "Queue Table Control"() -> (w84:string[][])
            n38 = Unbundle By Name(w82) -> ("Row"=w83:i32)  [unwired: 1 out]
            n39 = property on="Queue Table Control" class="Tbl (strict)"("Active Cell"=w82, "Cell BG Color"=u32 6618880 ("Active Cell:Cell Background Color")) -> ()  [unwired: 2 in, 2 out]
            n40 = Index Array(array=w84, index (row)=w83) -> (element=w80:string[])  [unwired: 1 in]
            n41 = local read "Queue Table"() -> (w78:string[][])
            n42 = Build Array (concatenate)(w78, w80) -> (w79:string[][])
            n43 = local write "Queue Table"(w79) -> ()
            n44 = call <vilib>:"Add State(s) to Queue__jki_lib_state_machine.vi"("State(s) in Front (\"\")"="Init: Queue Preset\nExpt Device Check>>Preset Queue", "State(s) in (\"\")"=w89) -> ("States Out"=w88:string)  [unwired: 13 in]
          }
          event "Queue Table": Mouse Down {
            n45 = event-data() -> ("Coords"=w92:T7, "Mods.Double Click"=w91:bool)  [unwired: 1 in, 6 out]
            n46 = case shown="True" w91 {
              tunnel: w92 -> [_ w110]
              frame False {
              }
              frame True {
                n47 = invoke on="Queue Table" class="Tbl (strict)" method="Point To Row Column"("Point"=w110) -> ("CellPosition"=w109:T2)  [unwired: 5 in, 5 out]
                n48 = Unbundle By Name(w109) -> ("Row"=w106:i32, "Column"=w105:i32)
                n49 = local read "Queue Table"() -> (w107:string[][])
                n50 = Delete From Array(array=w107, index (row)=w106) -> (array with subset deleted=w108:string[][])  [unwired: 2 in, 1 out]
                n51 = Index Array(array=w107, index (row)=w106, index (col)=w105) -> (element=w104:string)
                n52 = local read "Queue Table Control"() -> (w103:string[][])
                n53 = Index Array(array=w103, index (col)=0 ("disabled index (col)")) -> (element=w101:string[])  [unwired: 1 in]
                n54 = Search 1D Array(1D array=w101, element=w104) -> (index of element=w97:i32)  [unwired: 1 in]
                n55 = local write "Queue Table"(w108) -> ()
                n56 = Bundle By Name(cluster=T2 {"Row"=0, "Column"=0} ("Active Cell:Active Cell"), "Row"=w97) -> (w98:T2)
                n57 = property on="Queue Table Control" class="Tbl (strict)"("Active Cell"=w98, "Cell BG Color"=u32 16448250 ("Active Cell:Cell Background Color")) -> ()  [unwired: 2 in, 2 out]
              }
            }
            n58 = call <vilib>:"Add State(s) to Queue__jki_lib_state_machine.vi"("State(s) in (\"\")"=w95) -> ("States Out"=w94:string)  [unwired: 14 in]
          }
          event "Left Join": Value Change {
            n59 = event-data() -> ()  [unwired: 1 in, 6 out]
            n60 = call <vilib>:"Add State(s) to Queue__jki_lib_state_machine.vi"("State(s) in Front (\"\")"="Compare Table", "State(s) in (\"\")"=w113) -> ("States Out"=w112:string)  [unwired: 13 in]
          }
          event "Reset Queue": Value Change {
            n61 = event-data() -> ()  [unwired: 1 in, 6 out]
            n62 = call <vilib>:"Add State(s) to Queue__jki_lib_state_machine.vi"("State(s) in Front (\"\")"="Reset Queue", "State(s) in (\"\")"=w118) -> ("States Out"=w117:string)  [unwired: 13 in]
          }
          event "Choose Values": Value Change {
            (unwired) FALSE ("Choose Values")
            n63 = event-data() -> ()  [unwired: 1 in, 6 out]
            n64 = call <vilib>:"Add State(s) to Queue__jki_lib_state_machine.vi"("State(s) in Front (\"\")"="Choose Values", "State(s) in (\"\")"=w123) -> ("States Out"=w122:string)  [unwired: 13 in]
          }
          event "EXIT": Value Change {
            # "Exit Button Value Change (pressed) Event\n(this executes Macro: Exit to terminate the VI)"
            n65 = event-data() -> ()  [unwired: 1 in, 1 out]
            n66 = call <vilib>:"Add State(s) to Queue__jki_lib_state_machine.vi"("State(s) in Front (\"\")"="Macro: Exit", "State(s) in (\"\")"=w130) -> ("States Out"=w129:string)  [unwired: 13 in]
          }
          event Panel Close? {
            # "Discard the event because we'll close the front panel ourselves in Macro: Exit"
            # "Close Panel button (pressed) Event\n(this executes Macro: Exit to terminate the VI)"
            n67 = event-data() -> ()  [unwired: 1 in, 1 out]
            n68 = call <vilib>:"Add State(s) to Queue__jki_lib_state_machine.vi"("State(s) in Front (\"\")"="Macro: Exit", "State(s) in (\"\")"=w136) -> ("States Out"=w135:string)  [unwired: 13 in]
            n69 = event-data("Discard?"=TRUE) -> ()  [unwired: 1 in, 1 out]
          }
        }
      }
      frame "---------- Core ----------" {
        # "Do not put any code in this frame.\n(it is a separator no-op)"
        n70 = call <vilib>:"Add State(s) to Queue__jki_lib_state_machine.vi"("State(s) in (\"\")"=w140) -> ("States Out"=w139:string)  [unwired: 14 in]
      }
      frame Default {
        w150 = 42 items=["No error", "Argument error", "Memory is full", "Out of zone", "End of file", "File already open", "Generic file I/O error", "File not found", "File permission error", "Disk is full", "Duplicate path", "Too many files open", "System feature not enabled", "Resource file not found", "Cannot add resource", "Resource not found", "Image not found", "Image memory error", "Pen does not exist", "Config type invalid", "Config token not found", "Config parse error", "Config memory error", "Bad external code format", "Bad external code offset", "External code not present", "Null window", "Destroy window error", "Null menu", "Print aborted", "Bad print record", "Print driver error", "Windows error during printing", "Memory error during printing", "Print dialog error", "Generic print error", "Invalid device refnum", "Device not found", "Device parameter error", "Device unit error", "Cannot open device", "Device call aborted", "Generic error", "Cancelled by user", "Object ID too low", "Object ID too high", "Object not in heap", "Unknown heap", "Unknown object (invalid DefProc)", "Unknown object (DefProc not in table)", "Message out of range", "Invalid (null) method", "Unknown message", "Manager call not supported", "Bad address", "Network operation in progress", "Network operation timed out", "Connection is busy", "Network attribute not supported", "Network error", "Address in use", "System out of memory", "Connection aborted", "Connection refused", "Not connected", "Already connected", "Connection closed", "Initialization error (interapplication manager)", "Bad occurrence", "Wait on unbound occurrence handler", "Occurrence queue overflow", "Datalog type conflict", "Unused", "Unrecognized type (interapplication manager)", "Memory corrupt", "Failed to make temporary DLL", "Old CIN version", "Drag socket not found", "Failed to load drop-object", "Failed to register OLE object", "Failed to release OLE object", "Format specifier type mismatch", "Unknown format specifier", "Too few format specifiers", "Too many format specifiers", "Scan failed", "Newer CIN version", "Error converting to variant", "Runtime menu error", "Password tampered", "Variant attribute not found", "Incompatible variant data type", "Event data is not available", "Event Store is not present", "Occurrence is not found", "Event Queue is not created", "Event info is not available", "Refnum passed is NULL", "Error retrieving Class GUID", "Error retrieving CoClass GUID", "Error retrieving TypeLib GUID.", "Bad built application magic bytes.", "Specific driver is different from the specific driver associated with the Logical Name.", "There is no session opened to the class driver.", "Max Error", "MAX - Error with config objects", "MAX - Error loading configuration", "MAX - Group not supported"]
        # "Current State"
        # "Do not delete, rename, or modify this frame.\n(this is used to capture unhandled states and typos)"
        # "Handle mistyped state name (developer tool)"
        n71 = Format Into String(format string="Software Exception: Unhandled State \"%s\"." ("message"), error in=w146, w141) -> (resulting string=w149:string, error out=w148:errorcluster)  [unwired: 1 in]
        n72 = call <vilib>:"Error Cluster From Error Code.vi"("show call chain? (False)"=TRUE, "error in (no error)"=w148, "error message (\"\")"=w149, "error code (0)"=w150) -> ("error out"=w147:errorcluster)  [unwired: 5 in]
        n73 = call <vilib>:"Add State(s) to Queue__jki_lib_state_machine.vi"("State(s) in (\"\")"=w145) -> ("States Out"=w144:string)  [unwired: 14 in]
      }
      frame "Initialize Core Data" {
        # "Do not delete, rename, or modify this frame.\n(this is used to determine panel behavior on exit)"
        # "originally closed?"
        # "exe?"
        # "If panel starts closed or is an EXE, then close it when we exit"
        n74 = property class="VI"() -> ("FP.State"=w154:T4)  [unwired: 2 in, 2 out]
        n75 = property class="App"() -> ("App.Kind"=w160:T5)  [unwired: 2 in, 2 out]
        n76 = control-ref of="Current VI Reference"() -> (w155:refnum<vi>)
        n77 = Equal?(x=w154, y=T4."Closed" ("Front Panel Window:State")) -> (x = y?=w152:bool)
        n78 = Equal?(x=w160, y=T5."Run Time System" ("Application:Kind")) -> (x = y?=w158:bool)
        n79 = Or(x=w152, y=w158) -> (x .or. y?=w156:bool)
        n80 = Bundle By Name(cluster=w157, "Core.Current VI Reference"=w155, "Core.Close Panel on Exit?"=w156) -> (w162:T6)
        n81 = call <vilib>:"Add State(s) to Queue__jki_lib_state_machine.vi"("State(s) in (\"\")"=w164) -> ("States Out"=w163:string)  [unwired: 14 in]
      }
      frame "Error Handler" {
        # "Unhandled Error -- Display it"
        # "Handle any errors here.\nYou can also output any states to clean-up after errors occur"
        # "Clear error"
        n82 = call <vilib>:"General Error Handler.vi"("error in (no error)"=w166) -> ()  [unwired: 10 in, 5 out]
        n83 = call <vilib>:"Add State(s) to Queue__jki_lib_state_machine.vi"("State(s) in Front (\"\")"="/* Post Error States", "State(s) in (\"\")"=w170) -> ("States Out"=w169:string)  [unwired: 13 in]
      }
      frame "Exit" {
        # "Do not put any code in this frame.\n(No errors that occur here will be handled.)"
        n84 = call <vilib>:"Add State(s) to Queue__jki_lib_state_machine.vi"("State(s) in (\"\")"=w175) -> ("States Out"=w174:string)  [unwired: 14 in]
      }
      frame "---------- Data ----------" {
        # "Do not put any code in this frame.\n(It is a separator no-op. You can make a copy of this frame to create a new Data frame)"
        n85 = call <vilib>:"Add State(s) to Queue__jki_lib_state_machine.vi"("State(s) in (\"\")"=w179) -> ("States Out"=w178:string)  [unwired: 14 in]
      }
      frame "Data: Initialize" {
        w191 = T8 {"Current VI Reference"=refnum, "Close Panel on Exit?"=FALSE}  # Core
        w193 = TRUE  # Your Boolean data
        w192 = ""  # String
        # "do not delete - used by framework"
        # "Add new data here."
        # "Data names and types of shift register data are defined by this bundle."
        # "Initialize the shift-register data, here.\n(data names are defined by what you wire into the bundle function)"
        n86 = local read "Preset Table Control"() -> (w189:string[][])
        n87 = property on="Headers" class="Tbl (strict)"() -> ("Column Headers[]"=w190:string[])  [unwired: 2 in, 2 out]
        n88 = local read "Queue Table Control"() -> (w188:string[][])
        n89 = call "PresetExecutionDataCluster.vi"() -> ("Preset Manager Cluster"=w187:T9)  [unwired: 1 in]
        n90 = Bundle("Core"=w191, "Your Boolean data"=w193, "String"=w192, "Preset Table Control"=w189, "Column Headers[]"=w190, "Queue Table Control"=w188, "Preset Manager Cluster"=w187) -> (w186:T6)  [unwired: 1 in]
        n91 = call <vilib>:"Add State(s) to Queue__jki_lib_state_machine.vi"("State(s) in (\"\")"=w196) -> ("States Out"=w195:string)  [unwired: 14 in]
        n92 = Bundle By Name(cluster=w186, "Preset Manager Cluster.DevStatusQueue"="DevStatusQueue", "Preset Manager Cluster.Experiment Name"="Experiment Name", "Preset Manager Cluster.Software Root"="Software Root", "Preset Manager Cluster.Filtered Devices List"="Filtered Devices List", "Preset Manager Cluster.Virtual Devices List"="Virtual Devices List") -> (w185:T6)
      }
      frame "Data: Cleanup" {
        # "Cleanup any data and references, here.\n(this is called automatically, by the Macro: Exit)"
        n93 = Unbundle By Name(w197) -> ("Core.Current VI Reference"=w200:refnum<vi>)
        n94 = Close Reference(reference=w200, error in (no error)=w199) -> (error out=w198:errorcluster)
        n95 = call <vilib>:"Add State(s) to Queue__jki_lib_state_machine.vi"("State(s) in (\"\")"=w202) -> ("States Out"=w201:string)  [unwired: 14 in]
      }
      frame "---------- UI ----------" {
        # "Do not put any code in this frame.\n(It is a separator no-op. You can make a copy of this frame to create a new UI frame)"
        n96 = call <vilib>:"Add State(s) to Queue__jki_lib_state_machine.vi"("State(s) in (\"\")"=w206) -> ("States Out"=w205:string)  [unwired: 14 in]
      }
      frame "UI: Initialize" {
        # "Initialize the User Interface, here.\n(this is called automatically, by the Macro: Init)"
        n97 = call <vilib>:"Add State(s) to Queue__jki_lib_state_machine.vi"("State(s) in (\"\")"=w210) -> ("States Out"=w209:string)  [unwired: 14 in]
      }
      frame "UI: Cursor Set" {
        # "Argument"
        # "Set and Unset Cursor Busy.\n(Usage: \"UI: Cursor Set >> Busy|Idle\")"
        n98 = case shown="\"Idle\", Default" w211 {
          tunnel: w213 -> [w218 w220]
          tunnel: [w217 w219] -> w212
          frame "Idle", Default {
            n99 = call <vilib>:"Unset Busy.vi"("error in (no error)"=w218) -> ("error out"=w217:errorcluster)  [unwired: 10 in]
          }
          frame "Busy" {
            n100 = call <vilib>:"Set Busy.vi"("error in (no error)"=w220) -> ("error out"=w219:errorcluster)  [unwired: 9 in, 1 out]
          }
        }
        n101 = call <vilib>:"Add State(s) to Queue__jki_lib_state_machine.vi"("State(s) in (\"\")"=w216) -> ("States Out"=w215:string)  [unwired: 14 in]
      }
      frame "UI: Front Panel State" {
        # "Argument"
        # "Set Front Panel Open or Closed\n(Usage: \"UI: Front Panel State >> Open|Close\")"
        n102 = Unbundle By Name(w223) -> ("Core.Current VI Reference"=w222:refnum<vi>)
        n103 = case shown="\"Minimize\", \"Minimized\"" w221 {
          tunnel: w225 -> [w233 w248 w259 w272 w285]
          tunnel: [w235 w249 w261 w274 w287] -> w224
          tunnel: w222 -> [w234 w246 w260 w273 w286]
          frame "Open", "Standard", Default {
            w228 = T4."Standard" ("State")
            n104 = property class="VI"(reference=w234, error in=w233) -> (reference out=w231:refnum<vi>, error out=w232:errorcluster, "FP.State"=w230:T4)
            n105 = Not Equal?(x=w230, y=w228) -> (x != y?=w229:bool)
            n106 = case shown="True" w229 {
              tunnel: [w239 w241] -> w235
              tunnel: w232 -> [w238 w241]
              tunnel: w231 -> [w237 _]
              tunnel: w228 -> [w236 _]
              frame True {
                n107 = invoke class="VI" method="FP.Open"(reference=w237, error in=w238, "Activate"=TRUE, "State"=w236) -> (error out=w239:errorcluster)  [unwired: 1 in, 4 out]
              }
              frame False {
              }
            }
          }
          frame "Close", "Closed" {
            n108 = property class="VI"(reference=w246, error in=w248) -> (reference out=w245:refnum<vi>, error out=w247:errorcluster, "FP.State"=w243:T4)
            n109 = Not Equal?(x=w243, y=T4."Closed" ("Front Panel Window:State")) -> (x != y?=w242:bool)
            n110 = case shown="True" w242 {
              tunnel: [w250 w253] -> w249
              tunnel: w247 -> [w250 w252]
              tunnel: w245 -> [_ w251]
              frame False {
              }
              frame True {
                n111 = invoke class="VI" method="FP.Close"(reference=w251, error in=w252) -> (error out=w253:errorcluster)  [unwired: 1 in, 2 out]
              }
            }
          }
          frame "Hidden", "Hide" {
            w254 = T4."Hidden" ("State")
            n112 = property class="VI"(reference=w260, error in=w259) -> (reference out=w257:refnum<vi>, error out=w258:errorcluster, "FP.State"=w256:T4)
            n113 = Not Equal?(x=w256, y=w254) -> (x != y?=w255:bool)
            n114 = case shown="True" w255 {
              tunnel: [w265 w266] -> w261
              tunnel: w258 -> [w264 w266]
              tunnel: w257 -> [w263 _]
              tunnel: w254 -> [w262 _]
              frame True {
                n115 = invoke class="VI" method="FP.Open"(reference=w263, error in=w264, "State"=w262) -> (error out=w265:errorcluster)  [unwired: 2 in, 4 out]
              }
              frame False {
              }
            }
          }
          frame "Minimize", "Minimized" {
            w267 = T4."Minimized" ("State")
            n116 = property class="VI"(reference=w273, error in=w272) -> (reference out=w270:refnum<vi>, error out=w271:errorcluster, "FP.State"=w269:T4)
            n117 = Not Equal?(x=w269, y=w267) -> (x != y?=w268:bool)
            n118 = case shown="True" w268 {
              tunnel: [w278 w279] -> w274
              tunnel: w271 -> [w277 w279]
              tunnel: w270 -> [w276 _]
              tunnel: w267 -> [w275 _]
              frame True {
                n119 = invoke class="VI" method="FP.Open"(reference=w276, error in=w277, "State"=w275) -> (error out=w278:errorcluster)  [unwired: 2 in, 4 out]
              }
              frame False {
              }
            }
          }
          frame "Maximize", "Maximized" {
            w280 = T4."Maximized" ("State")
            n120 = property class="VI"(reference=w286, error in=w285) -> (reference out=w283:refnum<vi>, error out=w284:errorcluster, "FP.State"=w282:T4)
            n121 = Not Equal?(x=w282, y=w280) -> (x != y?=w281:bool)
            n122 = case shown="True" w281 {
              tunnel: [w291 w292] -> w287
              tunnel: w284 -> [w290 w292]
              tunnel: w283 -> [w289 _]
              tunnel: w280 -> [w288 _]
              frame True {
                n123 = invoke class="VI" method="FP.Open"(reference=w289, error in=w290, "State"=w288) -> (error out=w291:errorcluster)  [unwired: 2 in, 4 out]
              }
              frame False {
              }
            }
          }
        }
        n124 = call <vilib>:"Add State(s) to Queue__jki_lib_state_machine.vi"("State(s) in (\"\")"=w227) -> ("States Out"=w226:string)  [unwired: 14 in]
      }
      frame "---------- Macro ----------" {
        # "Do not put any code in this frame.\n(It is a separator no-op. You can make a copy of this frame to create a new Macro frame)"
        n125 = call <vilib>:"Add State(s) to Queue__jki_lib_state_machine.vi"("State(s) in (\"\")"=w296) -> ("States Out"=w295:string)  [unwired: 14 in]
      }
      frame "Macro: Initialize" {
        w300 = 0
        w299 = string[][] [] ("Queue Table")
        w303 = "Data: Initialize\nInitialize Core Data\nUI: Initialize\nUI: Front Panel State >> Open\nInitialize UDP Variables"  # Data: Initialize Initialize Core Data UI: Initialize UI: Front Panel State >> Open Initialize UDP Variables
        # "Initialization Macro\n(This is called once, when the VI starts)"
        n126 = property on="Queue Element" class="DigNum (strict)"("Value"=w300) -> ()  [unwired: 2 in, 2 out]
        n127 = property on="Queue Table" class="Tbl (strict)"("Value"=w299) -> ()  [unwired: 2 in, 2 out]
        n128 = property on="Queue Size" class="DigNum (strict)"("Value"=w300) -> ()  [unwired: 2 in, 2 out]
        n129 = property on="Preset Table Control" class="Tbl (strict)"("Value"=w299) -> ()  [unwired: 2 in, 2 out]
        n130 = property on="Preset Devices Not in Experiment" class="LstBox (strict)"("Item Names"=string[] [] ("Queue Table")) -> ()  [unwired: 2 in, 2 out]
        n131 = call <vilib>:"Add State(s) to Queue__jki_lib_state_machine.vi"("State(s) in Front (\"\")"=w303, "State(s) in (\"\")"=w307) -> ("States Out"=w306:string)  [unwired: 13 in]
        n132 = property on="Preset Execution Indicator" class="Bool (strict)"("Blinking"=FALSE, "Caption.Text"="" ("Boolean Text.Text"), "Colors [4]"=cluster{u32, u32}[] [{32639, 0}]) -> ()  [unwired: 2 in, 2 out]
      }
      frame "Macro: Exit" {
        # "Exit Macro\n(This is called once, when the VI exits)"
        n133 = Unbundle By Name(w314) -> ("Core.Close Panel on Exit?"=w313:bool)
        n134 = Select(t="UI: Front Panel State >> Close", s=w313, f="") -> (s? t:f=w310:string)
        n135 = call <vilib>:"Add State(s) to Queue__jki_lib_state_machine.vi"("State(s) in (\"\")"=w310, "State(s) at Back (\"\")"="Data: Cleanup\nExit") -> ("States Out"=w308:string)  [unwired: 13 in]
        n136 = call <vilib>:"Add State(s) to Queue__jki_lib_state_machine.vi"("State(s) in Front (\"\")"=w308, "State(s) in (\"\")"=w317) -> ("States Out"=w316:string)  [unwired: 13 in]
      }
      frame "Initialize UDP Variables" {
        # "Do not put any code in this frame.\n(It is a separator no-op. You can make a copy of this frame to create a new Macro frame)"
        n137 = Unbundle By Name(w326) -> ("Preset Manager Cluster.Experiment Name"=w324:string)
        n138 = call "UPD Variable Init.vi"("Expt Name"=w324) -> ("Mcast Address"=w320:string, "UDP timeout ms"=w321:i32, "MC Multicast"=w322:refnum<k16>, "My IP"=w323:string, "Mcast remote"=w319:u16, "> Name, devtype, ip, dev comm port, class, location for all devices>"=w318:string[][])  [unwired: 5 in]
        n139 = call <vilib>:"Add State(s) to Queue__jki_lib_state_machine.vi"("State(s) in (\"\")"=w329) -> ("States Out"=w328:string)  [unwired: 14 in]
        n140 = Bundle By Name(cluster=w326, "Preset Manager Cluster.My IP"=w323, "Preset Manager Cluster.MC Multicast"=w322, "Preset Manager Cluster.UDP timeout ms"=w321, "Preset Manager Cluster.Mcast address"=w320, "Preset Manager Cluster.MCast Remote"=w319, "Preset Manager Cluster.All Devices Core Info"=w318) -> (w325:T6)
      }
      frame "---------- Menu Control ----------" {
        # "Template Separator\n(You can make a copy of, or modify, this frame)"
        n141 = call <vilib>:"Add State(s) to Queue__jki_lib_state_machine.vi"("State(s) in (\"\")"=w333) -> ("States Out"=w332:string)  [unwired: 14 in]
      }
      frame "Compare Table" {
        # "Template Separator\n(You can make a copy of, or modify, this frame)"
        n142 = property on="PRESET FROM DB" class="Tbl (strict)"() -> ("Value"=w340:string[][])  [unwired: 2 in, 2 out]
        n143 = property on="ECS File" class="Tbl (strict)"() -> ("Value"=w339:string[][])  [unwired: 2 in, 2 out]
        n144 = call "Left Join.vi"("Array 2"=w339, "Array 1"=w340) -> ("Left Joined Array"=w337:string[][])  [unwired: 9 in]
        n145 = call <vilib>:"Add State(s) to Queue__jki_lib_state_machine.vi"("State(s) in Front (\"\")"="Table Update" ("State(s) in Front (\"\")"), "State(s) in (\"\")"=w343) -> ("States Out"=w342:string)  [unwired: 13 in]
        n146 = Bundle By Name(cluster=w338, "Preset Table Control"=w337, "Column Headers[]"=string[] ["Device Name", "Device Variable", "Preset Value", "ECS Value"] ("Column Headers")) -> (w336:T6)
      }
      frame "Choose Values" {
        # "Template Separator\n(You can make a copy of, or modify, this frame)"
        n147 = property on="Preset Table Control" class="Tbl (strict)"() -> ("Value"=w347:string[][])  [unwired: 2 in, 2 out]
        n148 = call "Value_Selection_in_Table_GUI.vi"("Column Headers"=string[] ["Device Name", "Device Variable", "Preset Value", "ECS Value"], "SELECTION TABLE - Click on values to keep"=w347) -> ("Coordinate Array"=→"Coordinate Array":i32[][])  [unwired: 9 in]
        n149 = call <vilib>:"Add State(s) to Queue__jki_lib_state_machine.vi"("State(s) in Front (\"\")"="Implement Value Change" ("State(s) in Front (\"\")"), "State(s) in (\"\")"=w351) -> ("States Out"=w350:string)  [unwired: 13 in]
      }
      frame "Implement Value Change" {
        # "Template Separator\n(You can make a copy of, or modify, this frame)"
        n150 = Unbundle By Name(w357) -> ("Preset Table Control"=w355:string[][])
        n151 = property on="Coordinate Array" class="Arr (strict)"() -> ("Value"=w354:i32[][])  [unwired: 2 in, 2 out]
        n152 = call "Value_Update_to_Preset.vi"("Coordinate Array with Changes"=w354, "Input Table"=w355) -> ("Column Headers"=w352:string[], "Output Table with Changes"=w353:string[][])  [unwired: 8 in]
        n153 = Bundle By Name(cluster=w357, "Preset Table Control"=w353, "Column Headers[]"=w352) -> (w356:T6)
        n154 = call <vilib>:"Add State(s) to Queue__jki_lib_state_machine.vi"("State(s) in Front (\"\")"="Table Update" ("State(s) in Front (\"\")"), "State(s) in (\"\")"=w361) -> ("States Out"=w360:string)  [unwired: 13 in]
      }
      frame "Load Preset from DB" {
        # "Template Separator\n(You can make a copy of, or modify, this frame)"
        n155 = property on="Preset Menu" class="Ring (strict)"() -> ("RingText.Text"=w362:string)  [unwired: 2 in, 2 out]
        n156 = call "Preset_to_Array.vi"("Preset Name"=w362) -> ("Column Headers"=w364:string[], "Preset Table"=w363:string[][])  [unwired: 9 in]
        "PRESET FROM DB" <- w363
        n157 = Bundle By Name(cluster=w367, "Preset Table Control"=w363, "Column Headers[]"=w364, "Preset Manager Cluster.PresetName"=w362) -> (w366:T6)
        n158 = call <vilib>:"Add State(s) to Queue__jki_lib_state_machine.vi"("State(s) in Front (\"\")"="Table Update\nExpt Device Check>>Preset Only" ("State(s) in Front (\"\")"), "State(s) in (\"\")"=w370) -> ("States Out"=w369:string)  [unwired: 13 in]
      }
      frame "Load Configuration File" {
        # "Template Separator\n(You can make a copy of, or modify, this frame)"
        n159 = call "Configuration_to_Array.vi"("file (use dialog)"="Navigate to ECS File") -> ("Table Control"=w373:string[][])  [unwired: 10 in]
        "ECS File" <- w373
        n160 = Bundle By Name(cluster=w375, "Preset Table Control"=w373, "Column Headers[]"=string[] ["Device Name", "Device Variable", "ECS Values"] ("Column Headers")) -> (w374:T6)
        n161 = call <vilib>:"Add State(s) to Queue__jki_lib_state_machine.vi"("State(s) in Front (\"\")"="Table Update" ("State(s) in Front (\"\")"), "State(s) in (\"\")"=w379) -> ("States Out"=w378:string)  [unwired: 13 in]
      }
      frame "Save Preset" {
        # "Template Separator\n(You can make a copy of, or modify, this frame)"
        n162 = call <vilib>:"Three Button Dialog.vi"("Right Button Text (\"Cancel\")"="Cancel" ("Right Button Text (\"Cancel\")"), "Center Button Text (\"No\")"="Overwrite Existing Preset" ("Right Button Text (\"Cancel\")"), "Left Button Text (\"Yes\")"="Save as New Preset" ("Left Button Text (\"Yes\")"), "message"="Save the current preset as - ") -> ("Which Button?"=w381:T10)  [unwired: 7 in]
        n163 = case shown="\"Right Button\", Default" w381 {
          tunnel: ["Save as New Preset" ("State(s) in Front (\"\")") "Overwrite Existing Preset" ("Right Button Text (\"Cancel\")") _] -> w380
          frame "Left Button" {
          }
          frame "Center Button" {
          }
          frame "Right Button", Default {
          }
        }
        n164 = call <vilib>:"Add State(s) to Queue__jki_lib_state_machine.vi"("State(s) in Front (\"\")"=w380, "State(s) in (\"\")"=w389) -> ("States Out"=w388:string)  [unwired: 13 in]
      }
      frame "Save as New Preset" {
        # "Template Separator\n(You can make a copy of, or modify, this frame)"
        n165 = call "Preset Name"() -> ("Name"=w393:string, "OK"=w402:bool)  [unwired: 17 in, 1 out]
        n166 = property on="Preset Menu" class="Ring (strict)"() -> ("Strings []"=w399:string[])  [unwired: 2 in, 2 out]
        n167 = Search 1D Array(1D array=w399, element=w393) -> (index of element=w398:i32)  [unwired: 1 in]
        n168 = call <vilib>:"Trim Whitespace.vi"("string"=w393) -> ("trimmed string"=w401:string)  [unwired: 1 in]
        n169 = Equal?(x=w401, y="") -> (x = y?=w396:bool)
        n170 = Not Equal?(x=w398, y=-1) -> (x != y?=w395:bool)
        n171 = Or(x=w396, y=w395) -> (x .or. y?=w394:bool)
        n172 = case shown="True" w402 {
          tunnel: w394 -> [_ w408]
          tunnel: w393 -> [_ w407]
          frame False {
          }
          frame True {
            n173 = case shown="False" w408 {
              tunnel: w407 -> [w409 _]
              frame False {
                n174 = stacked-sequence {
                  tunnel: w409 -> [w411]
                  frame #0 {
                    n175 = local read "Preset Table Control"() -> (w410:string[][])
                    n176 = for {
                      tunnel: w411 -> [w416]
                      tunnel: w410 -> [w412] mode=indexing
                      n177 = Insert Into Array(array=w412, index=0, new element=w416) -> (w414:string[])
                      n178 = call "SQL Insert null.vi"("Values"=w414, "Column Names"=string[] ["presetName", "presetDevice", "presetVariable", "presetValue"], "Table"="Presets") -> ("Query String"=w413:string)  [unwired: 8 in]
                      n179 = disable-structure shown="Enabled" {
                        disable-tunnel: w413 -> [w419 _]
                        frame Enabled {
                          n180 = call "SQL Server Info.vi"() -> ("SQL Server Info"=w420:T12)
                          n181 = call "SQL Query.vi"("SQL Server Info"=w420, "Query"=w419) -> ()  [unwired: 8 in, 2 out]
                        }
                        frame Disabled {
                        }
                      }
                    }
                  }
                }
              }
              frame True {
                n182 = One Button Dialog(message="Name field was blank or the Preset Name already exists") -> ()  [unwired: 1 in, 1 out]
              }
            }
          }
        }
        n183 = call <vilib>:"Add State(s) to Queue__jki_lib_state_machine.vi"("State(s) in Front (\"\")"="Load Preset from DB>>Table Update" ("State(s) in Front (\"\")"), "State(s) in (\"\")"=w406) -> ("States Out"=w405:string)  [unwired: 13 in]
      }
      frame "Overwrite Existing Preset" {
        # "Template Separator\n(You can make a copy of, or modify, this frame)"
        n184 = property on="Preset Menu" class="Ring (strict)"() -> ("RingText.Text"=w423:string)  [unwired: 2 in, 2 out]
        n185 = Concatenate Strings("Are you sure you want to overwrite " ("string"), w423, " with the current table ?" ("string")) -> (w426:string)
        n186 = Two Button Dialog(message=w426, 2:"Yes" ("T button name (\"OK\")")) -> (T button?=w424:bool)  [unwired: 1 in]
        n187 = case shown="True" w424 {
          tunnel: w423 -> [_ w433]
          frame False {
          }
          frame True {
            n188 = stacked-sequence {
              seq-local: [w434 _] -> [_ w444]
              tunnel: w433 -> [w435 w443]
              tunnel: [_ w444] -> _
              frame #0 {
                n189 = disable-structure shown="Enabled" {
                  disable-tunnel: w435 -> [w439 _]
                  disable-tunnel: [w436 _] -> w434
                  frame Enabled {
                    n190 = Concatenate Strings("DELETE FROM Presets WHERE presetName='", w439, "'" ("string")) -> (w437:string)
                    n191 = call "SQL Server Info.vi"() -> ("SQL Server Info"=w441:T12)
                    n192 = call "SQL Query.vi"("SQL Server Info"=w441, "Query"=w437) -> ("error out"=w436:errorcluster)  [unwired: 8 in, 1 out]
                  }
                  frame Disabled {
                  }
                }
              }
              frame #1 {
                n193 = local read "Preset Table Control"() -> (w442:string[][])
                n194 = for {
                  tunnel: w444 -> [w452]
                  tunnel: w443 -> [w449]
                  tunnel: w442 -> [w445] mode=indexing
                  n195 = Insert Into Array(array=w445, index=0, new element=w449) -> (w447:string[])
                  n196 = call "SQL Insert null.vi"("Values"=w447, "Column Names"=string[] ["presetName", "presetDevice", "presetVariable", "presetValue"], "Table"="Presets") -> ("Query String"=w446:string)  [unwired: 8 in]
                  n197 = disable-structure shown="Enabled" {
                    disable-tunnel: w452 -> [w454 _]
                    disable-tunnel: w446 -> [w453 _]
                    frame Enabled {
                      n198 = call "SQL Server Info.vi"() -> ("SQL Server Info"=w455:T12)
                      n199 = call "SQL Query.vi"("error in (no error)"=w454, "SQL Server Info"=w455, "Query"=w453) -> ()  [unwired: 7 in, 2 out]
                    }
                    frame Disabled {
                    }
                  }
                }
              }
            }
          }
        }
        n200 = call <vilib>:"Add State(s) to Queue__jki_lib_state_machine.vi"("State(s) in Front (\"\")"="Load Preset from DB>>Table Update" ("State(s) in Front (\"\")"), "State(s) in (\"\")"=w432) -> ("States Out"=w431:string)  [unwired: 13 in]
      }
      frame "Delete Preset" {
        # "Template Separator\n(You can make a copy of, or modify, this frame)"
        n201 = property on="Preset Menu" class="Ring (strict)"() -> ("RingText.Text"=w456:string)  [unwired: 2 in, 2 out]
        n202 = Concatenate Strings("Are you sure you want to delete " ("string"), w456, ". NOTE - THIS ACTION IS NOT REVERSIBLE" ("string")) -> (w459:string)
        n203 = Two Button Dialog(message=w459, 2:"Yes" ("T button name (\"OK\")")) -> (T button?=w457:bool)  [unwired: 1 in]
        n204 = case shown="True" w457 {
          tunnel: w456 -> [_ w467]
          frame False {
          }
          frame True {
            n205 = stacked-sequence {
              tunnel: w467 -> [w468]
              frame #0 {
                n206 = disable-structure shown="Disabled" {
                  disable-tunnel: w468 -> [w473 _]
                  frame Disabled {
                    n207 = Concatenate Strings("DELETE FROM Presets WHERE presetName='", w473, "'" ("string")) -> (w469:string)
                    n208 = call "SQL Server Info.vi"() -> ("SQL Server Info"=w472:T12)
                    n209 = call "SQL Query.vi"("SQL Server Info"=w472, "Query"=w469) -> ()  [unwired: 8 in, 2 out]
                  }
                  frame Enabled {
                  }
                }
              }
            }
          }
        }
        n210 = call <vilib>:"Add State(s) to Queue__jki_lib_state_machine.vi"("State(s) in Front (\"\")"="Load Preset from DB>>Table Update" ("State(s) in Front (\"\")"), "State(s) in (\"\")"=w466) -> ("States Out"=w465:string)  [unwired: 13 in]
      }
      frame "Execute Preset" {
        # "Template Separator\n(You can make a copy of, or modify, this frame)"
        n211 = property on="Preset Execution Indicator" class="Bool (strict)"("Blinking"=TRUE, "Caption.Text"="Executing Preset" ("Boolean Text.Text")) -> ()  [unwired: 2 in, 2 out]
        n212 = call <vilib>:"Add State(s) to Queue__jki_lib_state_machine.vi"("State(s) in Front (\"\")"="Send Preset Command" ("State(s) in Front (\"\")"), "State(s) in (\"\")"=w480) -> ("States Out"=w479:string)  [unwired: 13 in]
      }
      frame "-------Table Update--------" {
        # "Template Separator\n(You can make a copy of, or modify, this frame)"
        n213 = call <vilib>:"Add State(s) to Queue__jki_lib_state_machine.vi"("State(s) in (\"\")"=w484) -> ("States Out"=w483:string)  [unwired: 14 in]
      }
      frame "Table Update" {
        # "Template Separator\n(You can make a copy of, or modify, this frame)"
        n214 = Unbundle By Name(w487) -> ("Preset Table Control"=w486:string[][], "Column Headers[]"=w485:string[])
        n215 = call <vilib>:"Add State(s) to Queue__jki_lib_state_machine.vi"("State(s) in (\"\")"=w490) -> ("States Out"=w489:string)  [unwired: 14 in]
        n216 = property on="Preset Table Control" class="Tbl (strict)"("Value"=w486, "Column Headers[]"=w485) -> ()  [unwired: 2 in, 2 out]
      }
      frame "--------Queue Presets------------" {
        # "Template Separator\n(You can make a copy of, or modify, this frame)"
        n217 = call <vilib>:"Add State(s) to Queue__jki_lib_state_machine.vi"("State(s) in (\"\")"=w494) -> ("States Out"=w493:string)  [unwired: 14 in]
      }
      frame "Init: Queue Preset" {
        # "Template Separator\n(You can make a copy of, or modify, this frame)"
        n218 = property on="Tab Control" class="TabCtl (strict)"() -> ("Value"=w495:T1)  [unwired: 2 in, 2 out]
        n219 = Equal?(x=w495, y=1) -> (x = y?=w498:bool)
        n220 = case shown="False" w498 {
          frame False {
          }
          frame True {
            n221 = call "preset SQL Queries.vi"("Preset Query"=Preset_Query_Enum."GetAllPresetNames") -> ("data"=w502:string[][])  [unwired: 8 in, 2 out]
            n222 = Array Subset(array=w502, index (row)=1 ("index")) -> (w503:string[][])  [unwired: 3 in]
            n223 = property on="Queue Table Control" class="Tbl (strict)"("Value"=w503) -> ()  [unwired: 2 in, 2 out]
          }
        }
        n224 = call <vilib>:"Add State(s) to Queue__jki_lib_state_machine.vi"("State(s) in (\"\")"=w501) -> ("States Out"=w500:string)  [unwired: 14 in]
      }
      frame "Reset Queue" {
        # "Template Separator\n(You can make a copy of, or modify, this frame)"
        n225 = property on="Queue Table" class="Tbl (strict)"("Value"=string[][] [] ("Queue Table")) -> ()  [unwired: 2 in, 2 out]
        n226 = call <vilib>:"Add State(s) to Queue__jki_lib_state_machine.vi"("State(s) in (\"\")"=w510) -> ("States Out"=w509:string)  [unwired: 14 in]
      }
      frame "Execute Queue" {
        # "Template Separator\n(You can make a copy of, or modify, this frame)"
        n227 = flat-sequence {
          frame #0 {
            w516 = TRUE
            n228 = property on="Queue Progress Bar" class="Slide (strict)"("Visible"=w516) -> ()  [unwired: 2 in, 2 out]
            n229 = property on="Current Preset Queue Element" class="Str"("Visible"=w516) -> ()  [unwired: 2 in, 2 out]
            n230 = property on="Queue Size" class="DigNum (strict)"("Visible"=w516) -> ()  [unwired: 2 in, 2 out]
          }
          frame #1 {
            n231 = property on="Queue Table" class="Tbl (strict)"() -> ("Value"=w524:string[][])  [unwired: 2 in, 2 out]
            n232 = Index Array(array=w524, index (col)=0 ("disabled index (col)")) -> (element=w522:string[])  [unwired: 1 in]
            n233 = Array Size(array=w522) -> (size(s)=→"Queue Size":i32)
            n234 = property on="Using Queue" class="Bool (strict)"("Val(Sgnl)"=TRUE ("Value (Signaling)")) -> ()  [unwired: 2 in, 2 out]
            n235 = property on="Queue Progress Bar" class="Slide (strict)"("Value"=u8 0 ("Queue Progress Bar"), "Maximum"=1.0 ("Data Entry Limits:Maximum")) -> ()  [unwired: 2 in, 2 out]
            "Queue Element" <- 1 ("Element")
          }
          frame #2 {
          }
        }
        n236 = call <vilib>:"Add State(s) to Queue__jki_lib_state_machine.vi"("State(s) in Front (\"\")"="Preset Queue Loading" ("State(s) in Front (\"\")"), "State(s) in (\"\")"=w515) -> ("States Out"=w514:string)  [unwired: 13 in]
      }
      frame "Preset Queue Loading" {
        # "Template Separator\n(You can make a copy of, or modify, this frame)"
        n237 = flat-sequence {
          tunnel: w526 -> [w534]
          tunnel: [w535] -> w527
          tunnel: [w533] -> w525
          frame #0 {
            n238 = property on="Queue Element" class="DigNum (strict)"() -> ("Value"=w532:i32)  [unwired: 2 in, 2 out]
            n239 = property on="Queue Size" class="DigNum (strict)"() -> ("Value"=w531:i32)  [unwired: 2 in, 2 out]
            n240 = Less?(x=w531, y=w532) -> (x < y?=w536:bool)
            n241 = case shown="False" w536 {
              tunnel: [w542 ""] -> w535
              tunnel: w534 -> [w541 w552]
              tunnel: [w540 w552] -> w533
              tunnel: w532 -> [w539 _]
              tunnel: w531 -> [w538 _]
              frame False {
                n242 = Divide(x=w539, y=w538) -> (x/y=w537:dbl)
                n243 = flat-sequence {
                  tunnel: w541 -> [w545]
                  tunnel: [w544] -> w540
                  tunnel: ["Execute Preset"] -> w542
                  frame #0 {
                    n244 = property on="Queue Element" class="DigNum (strict)"() -> ("Value"=w547:i32)  [unwired: 2 in, 2 out]
                    n245 = local read "Queue Table"() -> (w549:string[][])
                    n246 = Decrement(x=w547) -> (x-1=w546:i32)
                    n247 = Index Array(array=w549, index (row)=w546, index (col)=0 ("disabled index (col)")) -> (element=w543:string)
                    "Current Preset Queue Element" <- w543
                    n248 = Bundle By Name(cluster=w545, "Preset Manager Cluster.PresetName"=w543) -> (w544:T6)
                  }
                  frame #1 {
                  }
                }
                n249 = property on="Queue Progress Bar" class="Slide (strict)"("Value"=w537) -> ()  [unwired: 2 in, 2 out]
              }
              frame True {
                n250 = property on="Using Queue" class="Bool (strict)"("Val(Sgnl)"=FALSE ("Value (Signaling)")) -> ()  [unwired: 2 in, 2 out]
              }
            }
          }
        }
        n251 = call <vilib>:"Add State(s) to Queue__jki_lib_state_machine.vi"("State(s) in Front (\"\")"=w527, "State(s) in (\"\")"=w530) -> ("States Out"=w529:string)  [unwired: 13 in]
      }
      frame "-------Preset Execution----------" {
        # "Template Separator\n(You can make a copy of, or modify, this frame)"
        n252 = call <vilib>:"Add State(s) to Queue__jki_lib_state_machine.vi"("State(s) in (\"\")"=w557) -> ("States Out"=w556:string)  [unwired: 14 in]
      }
      frame "MC Control Update" {
        # "Template Separator\n(You can make a copy of, or modify, this frame)"
        n253 = disable-structure shown="Disabled" {
          disable-tunnel: w559 -> [w570 w571]
          disable-tunnel: [w563 w571] -> w558
          frame Disabled {
            n254 = Bundle By Name(cluster=w570, "Preset Manager Cluster.My IP"="My IP", "Preset Manager Cluster.Mcast address"="Mcast address", "Preset Manager Cluster.MCast Remote"="MCast Remote", "Preset Manager Cluster.UDP timeout ms"="UDP timeout ms", "Preset Manager Cluster.MC Multicast"="MC Multicast", "Preset Manager Cluster.All Devices Core Info"="All Devices Core Info") -> (w563:T6)
          }
          frame Enabled {
          }
        }
        n255 = call <vilib>:"Add State(s) to Queue__jki_lib_state_machine.vi"("State(s) in (\"\")"=w562) -> ("States Out"=w561:string)  [unwired: 14 in]
      }
      frame "General wait" {
        # "Template Separator\n(You can make a copy of, or modify, this frame)"
        n256 = call "get arguments of jki state.vi"("jki arguments"=w572) -> ("Arg 1"=w574:string)  [unwired: 1 in, 2 out]
        n257 = Decimal String To Number(string=w574) -> (number=w573:i32)  [unwired: 2 in, 1 out]
        n258 = Wait (ms)(milliseconds to wait=w573) -> ()  [unwired: 1 out]
        n259 = call <vilib>:"Add State(s) to Queue__jki_lib_state_machine.vi"("State(s) in (\"\")"=w578) -> ("States Out"=w577:string)  [unwired: 14 in]
      }
      frame "Poll Devices" {
        # "rem virt devs"
        # "Template Separator\n(You can make a copy of, or modify, this frame)"
        n260 = Unbundle By Name(w597) -> ("Preset Manager Cluster"=w596:T9)
        n261 = Unbundle By Name(w596) -> ("PresetName"=w583:string, "Current Preset Devices"=w592:string[], "All Devices Core Info"=w595:string[][], "Filtered Devices List"=w594:string[], "Virtual Devices List"=w593:string[], "DevStatusQueue"=w587:refnum<queue>)
        n262 = Preview Queue Element(queue=w587, timeout in ms (-1)=200) -> (element=w586:string[][], error out=→"error out":errorcluster)  [unwired: 1 in, 2 out]
        n263 = call "search string array for elements in 2nd string array.vi"("search for"=w593, "search in"=w594) -> ("Indices of Elements"=w598:i32[])  [unwired: 9 in]
        n264 = call-poly <userlib>:"Delete Elements from Array__ogtk.vi"("indices"=w598, "array"=w594) -> ("array w/ subset deleted"=w589:string[])  [unwired: 8 in, 1 out]
        n265 = call "get info from core device data.vi"("devices to get data from"=w589, "All Devices Core Info"=w595) -> ("IP Addresses"=w590:string[])  [unwired: 2 in, 1 out]
        n266 = Empty Array?(array=w590) -> (empty?=w591:bool)
        n267 = flat-sequence {
          tunnel: w592 -> [w608]
          tunnel: w591 -> [w607]
          tunnel: w590 -> [w606]
          tunnel: w589 -> [w605]
          tunnel: w586 -> [w604]
          tunnel: w583 -> [w602]
          tunnel: [w602] -> w580
          tunnel: [w603] -> w581
          tunnel: [w630] -> w584
          tunnel: w581 -> [w630]
          tunnel: w580 -> [w624]
          tunnel: [w623] -> w579
          frame #0 {
            n268 = case shown="False" w607 {
              tunnel: w602 -> [w615 _]
              tunnel: w608 -> [w614 _]
              tunnel: w606 -> [w613 _]
              tunnel: w605 -> [w612 _]
              tunnel: w604 -> [w610 _]
              tunnel: [w609 FALSE ("Active Preset Achieved")] -> w603
              frame False {
                # "Determine which devices are ON/OFF"
                n269 = call "get device status from tcp data array.vi"("TCP Device status data"=w610, "Current Preset Devices"=w614, "IP Addresses in"=w613, "Filtered Device List"=w612, "Requested Preset"=w615) -> ("Device Errors"=→"Device Errors":string[][], "Active boolean array"=→"Active Device array":bool[], "preset diagnostics"=w616:T13, "Active IP Addresses"=→"Active Dev/IP":string[], "Devices Not alive"=→"Devices not started":string[])  [unwired: 3 in, 3 out]
                n270 = Unbundle By Name(w616) -> ("Active Preset Achieved"=w609:bool)
                n271 = Select(t=w615, s=w609, f="Undefined") -> (s? t:f=→"Active Preset":string)
              }
              frame True {
              }
            }
          }
          frame #1 {
            n272 = property on="Active Preset" class="Str"() -> ("Value"=w626:string)  [unwired: 2 in, 2 out]
            n273 = property on="Poll Count" class="DigNum (strict)"() -> ("Value"=w628:i32)  [unwired: 2 in, 2 out]
            n274 = Not Equal?(x=w624, y=w626) -> (x != y?=w627:bool)
            n275 = Less?(x=w628, y=8) -> (x < y?=w629:bool)
            n276 = And(x=w627, y=w629) -> (x .and. y?=w623:bool)
          }
        }
        n277 = case shown="True" w579 {
          tunnel: w584 -> [w632 _]
          tunnel: [w631 "General Wait>>3000\nPoll Devices"] -> w582
          frame False {
            n278 = case shown="True" w632 {
              tunnel: ["" w638] -> w631
              frame False {
                n279 = property on="Preset Execution Indicator" class="Bool (strict)"("Blinking"=FALSE, "Caption.Text"=" Preset Failed" ("Boolean Text.Text"), "Value"=FALSE ("Blinking"), "Colors [4]"=cluster{u32, u32}[] [{16711680, 0}]) -> ()  [unwired: 2 in, 2 out]
              }
              frame True {
                n280 = property on="Using Queue" class="Bool (strict)"() -> ("Value"=w639:bool)  [unwired: 2 in, 2 out]
                n281 = property on="Preset Execution Indicator" class="Bool (strict)"("Blinking"=FALSE, "Caption.Text"=" Preset Executed" ("Boolean Text.Text"), "Value"=TRUE ("Blinking"), "Colors [4]"=cluster{u32, u32}[] [{318464, 0}]) -> ()  [unwired: 2 in, 2 out]
                n282 = case shown="False" w639 {
                  tunnel: ["" "Preset Queue Loading"] -> w638
                  frame False {
                  }
                  frame True {
                    n283 = property on="Queue Element" class="DigNum (strict)"() -> ("Value"=w647:i32)  [unwired: 2 in, 2 out]
                    n284 = Increment(x=w647) -> (x+1=w646:i32)
                    n285 = property on="Queue Element" class="DigNum (strict)"("Value"=w646) -> ()  [unwired: 2 in, 2 out]
                  }
                }
              }
            }
          }
          frame True {
            n286 = property on="Poll Count" class="DigNum (strict)"() -> ("Value"=w650:i32)  [unwired: 2 in, 2 out]
            n287 = Increment(x=w650) -> (x+1=w649:i32)
            n288 = property on="Poll Count" class="DigNum (strict)"("Value"=w649) -> ()  [unwired: 2 in, 2 out]
          }
        }
        n289 = call <vilib>:"Add State(s) to Queue__jki_lib_state_machine.vi"("State(s) in Front (\"\")"=w582, "State(s) in (\"\")"=w601) -> ("States Out"=w600:string)  [unwired: 13 in]
      }
      frame "Send Preset Command" {
        # "This State builds the Multicast Preset Command to all Devices"
        # "Template Separator\n(You can make a copy of, or modify, this frame)"
        n290 = Unbundle By Name(w657) -> ("Preset Manager Cluster.My IP"=w656:string, "Preset Manager Cluster.PresetName"=w652:string)
        n291 = call "preset SQL Queries.vi"("Expt name / MCIP/ Variable/Preset Name"=w652, "Preset Query"=Preset_Query_Enum."GetPresetDeviceNames") -> ("1st column 1st data"=w654:string[])  [unwired: 7 in, 2 out]
        n292 = Concatenate Strings("preset>>" ("string"), w652, ">>" ("string"), w656) -> (w655:string)
        n293 = Bundle By Name(cluster=w657, "Preset Manager Cluster.PresetName"=w652, "Preset Manager Cluster.Mcast command"=w655, "Preset Manager Cluster.Current Preset Devices"=w654) -> (w658:T6)
        n294 = property on="Poll Count" class="DigNum (strict)"("Value"=0) -> ()  [unwired: 2 in, 2 out]
        n295 = call <vilib>:"Add State(s) to Queue__jki_lib_state_machine.vi"("State(s) in (\"\")"=w664, "State(s) at Back (\"\")"="Send Multicast>>Empty\nGeneral wait>>10\nSend Multicast>>Empty\nGeneral wait>>40\nSend Multicast\nGeneral wait>>3000\nPoll Devices" ("Remaining States")) -> ("States Out"=w663:string)  [unwired: 13 in]
      }
      frame "Send Multicast" {
        # "Template Separator\n(You can make a copy of, or modify, this frame)"
        n296 = Unbundle By Name(w667) -> ("Preset Manager Cluster.MCast Remote"=w673:u16, "Preset Manager Cluster.Mcast address"=w672:string, "Preset Manager Cluster.UDP timeout ms"=w670:i32, "Preset Manager Cluster.Mcast command"=w669:string, "Preset Manager Cluster.MC Multicast"=w668:refnum<k16>)
        n297 = String To IP(1:w672) -> (0:w671:u32)
        n298 = UDP Write(address=w671, port or service name=w673, connection ID=w668, data in=w669, 9:w670) -> (3:w665:refnum<k16>)  [unwired: 1 in, 1 out]
        n299 = Bundle By Name(cluster=w667, "Preset Manager Cluster.MC Multicast"=w665) -> (w666:T6)
        n300 = call <vilib>:"Add State(s) to Queue__jki_lib_state_machine.vi"("State(s) in (\"\")"=w676) -> ("States Out"=w675:string)  [unwired: 14 in]
      }
      frame "-------------Diagnostics-----------" {
        # "Template Separator\n(You can make a copy of, or modify, this frame)"
        n301 = call <vilib>:"Add State(s) to Queue__jki_lib_state_machine.vi"("State(s) in (\"\")"=w680) -> ("States Out"=w679:string)  [unwired: 14 in]
      }
      frame "Expt Device Check" {
        # "Template Separator\n(You can make a copy of, or modify, this frame)"
        n302 = Unbundle By Name(w694) -> ("Preset Manager Cluster.Experiment Name"=w684:string, "Preset Manager Cluster.PresetName"=w693:string, "Preset Manager Cluster.All Devices Core Info"=w683:string[][], "Preset Manager Cluster.DevStatusQueue"=w682:refnum<queue>)
        n303 = Equal?(x=w688, y="Preset Only") -> (x = y?=w687:bool)
        n304 = case shown="True" w687 {
          tunnel: [enum16{"Preset Queue", "Preset Only"}."Preset Queue" ("Input Type") enum16{"Preset Queue", "Preset Only"}."Preset Only" ("Input Type")] -> w686
          frame False {
          }
          frame True {
          }
        }
        n305 = property on="Queue Table" class="Tbl (strict)"() -> ("Value"=w685:string[][])  [unwired: 2 in, 2 out]
        n306 = call "Preset Expt Device Comparison.vi"("Input Type"=w686, "Preset Name"=w693, "Preset Array"=w685, "Expt name"=w684) -> ("Devices Not in Experiment"=w690:string[], "Devices accounted for?"=w692:bool)  [unwired: 6 in]
        n307 = property on="Preset Devices Not in Experiment" class="LstBox (strict)"("Item Names"=w690) -> ()  [unwired: 2 in, 2 out]
        n308 = call "Devices Not On.vi"("All Devices Core Info"=w683, "Experiment"=w684, "queue"=w682) -> ("Devices Not alive"=w681:string[])  [unwired: 8 in]
        n309 = property on="Expt Devices Not On" class="LstBox (strict)"("Item Names"=w681) -> ()  [unwired: 2 in, 2 out]
        n310 = case shown="True" w692 {
          tunnel: ["" ""] -> w691
          frame False {
            n311 = property on="Preset Execution Indicator" class="Bool (strict)"("Blinking"=FALSE, "Caption.Text"="Devices Not \nin Experiment" ("Boolean Text.Text"), "Value"=FALSE ("Blinking"), "Colors [4]"=cluster{u32, u32}[] [{16711680, 0}]) -> ()  [unwired: 2 in, 2 out]
          }
          frame True {
          }
        }
        n312 = call <vilib>:"Add State(s) to Queue__jki_lib_state_machine.vi"("State(s) in Front (\"\")"=w691, "State(s) in (\"\")"=w697) -> ("States Out"=w696:string)  [unwired: 13 in]
      }
      frame "Check Expt Device On" {
        # "Template Separator\n(You can make a copy of, or modify, this frame)"
        n313 = Unbundle By Name(w710) -> ("Preset Manager Cluster.Experiment Name"=w709:string, "Preset Manager Cluster.All Devices Core Info"=w708:string[][], "Preset Manager Cluster.DevStatusQueue"=w707:refnum<queue>)  [unwired: 1 out]
        n314 = call "Devices Not On.vi"("All Devices Core Info"=w708, "Experiment"=w709, "queue"=w707) -> ("Devices Not alive"=w706:string[])  [unwired: 8 in]
        n315 = property on="Expt Devices Not On" class="LstBox (strict)"("Item Names"=w706) -> ()  [unwired: 2 in, 2 out]
        n316 = call <vilib>:"Add State(s) to Queue__jki_lib_state_machine.vi"("State(s) in (\"\")"=w713) -> ("States Out"=w712:string)  [unwired: 14 in]
      }
    }
  }
